vi "PAHS Main.vi"() -> ()   [LabVIEW 2016]
uses:
  Libraries/Controls/Aux CO2 Diags.ctl
  Libraries/Controls/Aux CO2 Selector.ctl
  Libraries/Controls/Processed Variables.ctl
  Libraries/Controls/AirPump Controls.ctl
  Libraries/Controls/Hobbs Meter.ctl
  Libraries/Controls/DAQ Needed.ctl
  Libraries/Controls/IE Ratio knob.ctl
  Libraries/Controls/UI Settings.ctl
  Libraries/Controls/Aux CO2 Control.ctl
  Libraries/Controls/Serial Visa Control.ctl
  Libraries/Controls/Aux TE Control.ctl
  Libraries/Controls/Queues And Others.ctl
  Libraries/Controls/Temperature Cycle.ctl
  Libraries/Controls/Temperature Source.ctl
  <vilib>/Platform/TimedLoop/XDataNode/timing_clust.ctl
  <vilib>/Platform/TimedLoop/XDataNode/nitl_modes.ctl
  <vilib>/Platform/TimedLoop/XDataNode/wakeup.ctl
  Libraries/Miscellaneous/Globals.vi
  <vilib>/platform/TimedLoop/XDataNode/XDataNode.xnode
  <vilib>/Platform/TimedLoop/XDataNode/XDNodeRunTimeDep.lvlib
panel:
  in  "RunTime Mode Settings  2":T1={"Resp Rate Brpm "=0.0, "I:E Ratio"=6, "Insp. Gas Tank"=0, "Exp. Gas Tank"=7} {"Exp. Gas Tank" items=["", "0.000", "0.000", "0.000", "0.000", "0.000", "0.000", "0.000"]; "Insp. Gas Tank" items=["", "0.000", "0.000", "0.000", "0.000", "0.000", "0.000", "0.000"]; "I:E Ratio" max=7 step=1 scale=0.0..7.0; "Resp Rate Brpm" min=0 max=30 step=1 format="%.2f"}
  in  "Cluster 12":T2 {"DAC Setting (ma)" max=1023.0 step=1.0 format="%.2g"; "DAC Setting" max=1023 step=1 format="%02x"}
  out "Status Lights":T3
  in  "Daq Needed":T4 {"Current Settings"."Pump" items=["Pump 0", "Pump 1", "Pump 2", "Pump 3", "Pump 4", "Pump 5"]; "Current Settings"."Chart X axis Timescale" min=20 max=180 step=1; "Current Settings"."RunTime Mode Settings"."Exp. Gas Tank" items=["0.07", "0.031", "0.877", "1.863", "3.881", "5.790", "7.688", "6.000"]; "Current Settings"."RunTime Mode Settings"."Insp. Gas Tank" items=["0.07", "0.031", "0.877", "1.863", "3.881", "5.790", "7.688", "6.000"]; "Current Settings"."RunTime Mode Settings"."I:E Ratio" max=30 scale=0.0..7.0; "Current Settings"."RunTime Mode Settings"."Resp Rate Brpm" min=0 max=30 format="%.2f"; "Current Settings"."TE#2 Configuration"."Serial Port"."XOFF Char" format="%.0x"; "Current Settings"."TE#2 Configuration"."Serial Port"."XON Char" format="%.0x"; "Current Settings"."TE#2 Configuration"."Serial Port"."flow control" items=["None"=0, "XON/XOFF"=1, "RTS/CTS"=2, "DTR/DSR"=4]; "Current Settings"."TE#2 Configuration"."Serial Port"."stop bits" items=["1.0"=10, "1.5"=15, "2.0"=20]; "Current Settings"."TE#2 Configuration"."Serial Port"."data bits" min=5 max=8 step=1; "Current Settings"."TE#2 Configuration"."Serial Port"."baud rate" items=["75"=75, "110"=110, "134"=134, "150"=150, "300"=300, "600"=600, "1200"=1200, "1800"=1800, "2400"=2400, "4800"=4800, "7200"=7200, "9600"=9600, "14400"=14400, "19200"=19200, "28800"=28800, "38400"=38400, "56000"=56000, "57600"=57600, "115200"=115200, "128000"=128000, "230400"=230400]; "Current Settings"."TE#2 Configuration"."Serial Port"."termination char" format="%.0x"; "Current Settings"."TE#1 Configuration"."Serial Port"."XOFF Char" format="%.0x"; "Current Settings"."TE#1 Configuration"."Serial Port"."XON Char" format="%.0x"; "Current Settings"."TE#1 Configuration"."Serial Port"."flow control" items=["None"=0, "XON/XOFF"=1, "RTS/CTS"=2, "DTR/DSR"=4]; "Current Settings"."TE#1 Configuration"."Serial Port"."stop bits" items=["1.0"=10, "1.5"=15, "2.0"=20]; "Current Settings"."TE#1 Configuration"."Serial Port"."data bits" min=5 max=8 step=1; "Current Settings"."TE#1 Configuration"."Serial Port"."baud rate" items=["75"=75, "110"=110, "134"=134, "150"=150, "300"=300, "600"=600, "1200"=1200, "1800"=1800, "2400"=2400, "4800"=4800, "7200"=7200, "9600"=9600, "14400"=14400, "19200"=19200, "28800"=28800, "38400"=38400, "56000"=56000, "57600"=57600, "115200"=115200, "128000"=128000, "230400"=230400]; "Current Settings"."TE#1 Configuration"."Serial Port"."termination char" format="%.0x"; "Current Settings"."Capnometer Configuration"."Device" items=["None", "TidalWave", "LoFlow / Canary", "Capnogard"]; "Current Settings"."Capnometer Configuration"."Serial Port"."XOFF Char" format="%.0x"; "Current Settings"."Capnometer Configuration"."Serial Port"."XON Char" format="%.0x"; "Current Settings"."Capnometer Configuration"."Serial Port"."flow control" items=["None"=0, "XON/XOFF"=1, "RTS/CTS"=2, "DTR/DSR"=4]; "Current Settings"."Capnometer Configuration"."Serial Port"."stop bits" items=["1.0"=10, "1.5"=15, "2.0"=20]; "Current Settings"."Capnometer Configuration"."Serial Port"."data bits" min=5 max=8 step=1; "Current Settings"."Capnometer Configuration"."Serial Port"."baud rate" items=["75"=75, "110"=110, "134"=134, "150"=150, "300"=300, "600"=600, "1200"=1200, "1800"=1800, "2400"=2400, "4800"=4800, "7200"=7200, "9600"=9600, "14400"=14400, "19200"=19200, "28800"=28800, "38400"=38400, "56000"=56000, "57600"=57600, "115200"=115200, "128000"=128000, "230400"=230400]; "Current Settings"."Capnometer Configuration"."Serial Port"."termination char" format="%.0x"; "Current Settings"."DAQx Settings"."Analog Output Settings (Volts)" format="%#.3g"; "Current Settings"."DAQx Settings"."Duty Cycle" min=10.0 max=90.0 format="%.1g"; "Current Settings"."DAQx Settings"."Frequency" min=20.0 max=200.0; "Current Settings"."DataLogging Settings"."Data File Duration (Minutes)" min=2 max=200 format="%#.2g"; "Current Settings"."Calibration Settings"."Tolerance #2" min=2 max=4096; "Current Settings"."Calibration Settings"."Cal. Average" min=2 max=4096; "Current Settings"."Test Settings"."Test Sensor ID" items=["(select)", "RB", "YC", "", "Other"]}
  out "InitializeFile":bool caption="Reset"
  out "Ready":bool caption="Saving Data"
  out "Saving":bool
  in  "Prefix":string
  out "Humidity Error":bool
  out "BD":i32
  in  "breath start time":u32
  out "Raws":T12 {"Chamber Temperature" format="%.2f"; "Ambient Temperature" format="%.2f"; "Bath Temperature" format="%.2f"; "Det. Temperature" format="%.2f"; "Detector Chl 4" format="%.2g"; "Detector Chl 3" format="%.2g"; "Ref CO2" format="%.2g"; "Detector Chl 2" format="%.2g"; "Film Temperature" format="%.2f"; "Humidity" format="%.2f"; "Detector Chl 1" format="%.2g"}
  in  "Raw DAQ Channels 2":cluster{"String":string, "Value":sgl[]}[](array[cluster])=[{"String"="Detector Chnl 1", "Value"=[10.2235565]}, {"String"="Detector Chnl 2", "Value"=[10.219611]}, {"String"="Detector Chnl 3", "Value"=[10.215665]}, {"String"="Detector Chnl 4", "Value"=[10.196594]}, {"String"="CH AI1 - Temp", "Value"=[]}, {"String"="CH AI2 - Temp", "Value"=[]}, {"String"="CH AI3 - (spare)", "Value"=[]}, {"String"="CH AI4 - (spare)", "Value"=[]}, {"String"="CH AI5 - (spare)", "Value"=[]}, {"String"="CH AI6 - PHAvset", "Value"=[]}, {"String"="CH AI7 - PHBvset", "Value"=[]}, {"String"="CH AI8 - PHCvset", "Value"=[]}, {"String"="CH AI9 - PHDvset", "Value"=[]}] {"Value" format="%7.3f"}
  out "start mS time":u32
  in  "Insp Tank":u8
  out "sequence":i64[](array[numeric])
  out "TE Data":sgl[][](array[numeric]) format="%.2g"
  out "Exp Tank":u8
  in  "ExitProgram":bool
  out "Tab Control":T13(tab)
  out "Saving Data":bool
  in  "HomeMode":T14(tab) caption="Status"
  in  "Open Cal":bool
  in  "Store_Cal":bool
  out "Time Since last Zero":u32 format="%<%H:%M:%S>t"
  out "Time Since last Cal":u32 format="%<%H:%M:%S>t"
  in  "Record Button":bool
  out "Saving File":path
  out "starttime":u32
  in  "Zero 2":bool
  in  "Last Calibration":T15
  out "Monitoring Time since last Zero":dbl format="%<%H:%M:%S>t"
  in  "Cluster 3":T17={"pk"=0.0, "RawCO2"=0.0, "Uncal'd"=0.0, "Avg_Hum"=0.0, "Avg'd CO2"=0.0, "Home_CO2"=0.0, "Home_Ref"=0.0, "Home_Hum"=0.0, " Home Temp"=0.0, "Pump Flow Rate"=50, "I:E Ratio"=6, "Brpm"=6.0, "Sim Breaths"=FALSE, "GasTank"=0} {"Brpm" format="%#_2g"; "I:E Ratio" max=7 step=1 scale=0.0..7.0; "Pump Flow Rate" min=50 max=650 step=10 scale=50.0..650.0; "Home Temp" format="%.1f"; "Home_Hum" format="%.1f"; "Home_Ref" format="%.2g"; "Home_CO2" format="%.2g"; "Avg'd CO2" format="%.1g"; "Avg_Hum" format="%.1f"; "Uncal'd" format="%.1g"; "RawCO2" format="%.2g"; "pk" format="%.1g"}
  out "Zero Status":u16(ring)
  out "target":dbl=0.001
  out "standard deviation":u8(slide) scale=1.0..99.0
  out "zcount":i32(slide)=200 scale=0.0..500.0
  out "raws(V)":sgl[](array[numeric])
  out "Capnogram":dbl[][](graph)
  in  "Off":bool
  in  "Cal Required":bool
  in  "Zero Required":bool
  in  "Cluster 8":T18={"Display Uncal'd"=FALSE, "Display Ref"=FALSE, "Ch 1"=FALSE, "Ch 2"=FALSE, "Ch 3"=FALSE, "Ch 4"=TRUE}
  in  "Cluster 7":T19 {"Time Remaining" format="%<%H:%M:%S>t"; "File Duration" format="%<%H:%M:%S>t"}
  out "Char Notice":string="NOT AVAILABLE IN CHARACTERIZATION MODE"
  out "CalTab":enum32{"Page 2", "Page 1"}(tab)
  in  "Cluster 6":T21 {"Time" format="%<%H:%M:%S>t"; "Stable Counter" format="%<%H:%M:%S>t"; "Actual" format="%.2g"; "Set Temp" format="%#.2g"}
  in  "Cluster 5":T22={"ETCO2 %"=0.0, "RR (brpm)"=0.0, "Inhale Time"=0.0, "Exhale Time"=0.0, "Enable Simulated Breaths"=FALSE, "Use Channel"=4} {"Use Channel" min=1 max=4; "RR (brpm)" format="%#.1f"; "ETCO2 %" format="%.1f"}
  out "Waveform Chart 2":dbl[][](graph) caption="Waveform Chart"
  out "Waveform Chart":dbl[][](graph)
  in  "Waveforms":T23={"WaveformA1"=enum."CO2 Ch1", "WaveformA1"=enum."CO2 Ch2", "WaveformA1"=enum."CO2 Ch3", "WaveformA1"=enum."CO2 Ch4", "WaveformA1"=enum."Temp", "WaveformA1"=enum."Humidity", "WaveformA1"=enum."Ref CO2", "WaveformA1"=enum."TE 1&2"}
  out "Gas Tank#":u16(ring) items=["0.07", "0.030", "0.877", "1.863", "3.881", "5.900", "7.688", "6.000", "<OFF>"]
  out "Loflo Status":T24(ring)
  out "Film Sample Name":string
  out "Tank":bool[](array[boolean])
  out "Cluster 4":T25 {"Chamber C" format="%.2f"; "Ambient" format="%.2f"; "Det. `C" format="%.2f"; "Bath `C" format="%.2f"; "Film `C" format="%.2f"; "TE #2" format="%.2f"; "TE #1" format="%.2f"; "Humidity" format="%.2f"; "Ref CO2" format="%.2g"}
  out "Detector Channels":T26 {"Chl 4 (V)" format="%.3g"; "Chl 3 (V)" format="%.3g"; "Chl 2 (V)" format="%.3g"; "Chl 1 (V)" format="%.3g"; "CO2% (4)" format="%.2g"; "CO2% (3)" format="%.2g"; "CO2% (2)" format="%.2g"; "CO2% (1)" format="%.2g"}
  in  "Cluster 9":T27 {"Sensor Under Test" items=["(select)", "RB", "YC", "", "Other"]}
  in  "Cluster 2":T29={" Chamber Temp"=0.0, "Source"=enum."PCB (AI1)", "Bath Source"=TRUE} {"Chamber Temp" format="%.2f"}
  in  "Logging":T30={"Data File Path"=path "c:/data", "Log Filename"=path "", "Data File Duration (Minutes)"=2.0} {"Data File Duration (Minutes)" min=2 max=200 format="%#.2g"}
  out "Pump":u16(ring) items=["Pump 0", "Pump 1", "Pump 2", "Pump 3", "Pump 4", "Pump 5"]
  out "Pump Meter Use (mins)":T31 {"secs" format="%01d"; "mins" format="%01d"}
  in  "Offset Adjust":bool=TRUE
  out "DAC return":sgl[](array[numeric]) caption="Return" format="%.4f"
  out "System #":string
  in  "LEDsON":bool=TRUE
  out "main loop rate":sgl caption="Hz"
  in  "Humidifier":bool=TRUE
  in  "SetDac Button":bool
  in  "Zero":bool
  out "Ticks Interval Time":dbl(graph)
  out "TE Ports":T32 {"ProcessedData" format="%.2g"}
  out "Aux CO2 Port":T33={"Port"="", "Source"=0, "Active"=FALSE, "Baro Pressure"=760, "SerialRxBuffer"="", "Raw CO2 (Torr)"=5.0, "bytes read"=5, "Status"=[], "Status Message"=enum.""} {"Status" format="%x"; "Raw CO2 (Torr)" format="%.2f"; "Baro Pressure" min=400 max=800; "Source" items=["None", "TidalWave", "LoFlow / Canary", "Capnogard"]}
  out "stored time":dbl format="%<%H:%M:%S>t"
  out "stop time":timestamp format="%<%H:%M:%S>T"
  out "DAQ Raw Samples":waveform(dbl)(graph)
  out "loop counter":i32
  out "current time":timestamp format="%<%H:%M:%S>T"
  in  "Run":bool
  out "start time":timestamp format="%<%H:%M:%S>T"
  out "Notes":string
  out "Raw (Torr)":sgl=5.0
  out "Digital Output":T34(array[cluster])=[{"Boolean"=TRUE, "String"="PO.0", "String 2"="Test"}, {"Boolean"=FALSE, "String"="PO.1", "String 2"="Dual Channel"}, {"Boolean"=TRUE, "String"="PO.2", "String 2"="Air Pump"}, {"Boolean"=FALSE, "String"="PO.3", "String 2"="Optical Drive"}, {"Boolean"=TRUE, "String"="PO.4", "String 2"="Pulsed Drive"}, {"Boolean"=FALSE, "String"="PO.5", "String 2"="Exp. Phase"}, {"Boolean"=FALSE, "String"="PO.6", "String 2"="/Expiratory"}, {"Boolean"=FALSE, "String"="PO.7", "String 2"="Insp. Phase"}, {"Boolean"=FALSE, "String"="PO.8", "String 2"="/Inspiratory"}, {"Boolean"=TRUE, "String"="PO.9", "String 2"="Gas Tank #0"}, {"Boolean"=FALSE, "String"="PO.10", "String 2"="Gas Tank #1"}, {"Boolean"=FALSE, "String"="PO.11", "String 2"="Gas Tank #2"}, {"Boolean"=FALSE, "String"="PO.12", "String 2"="Gas Tank #3"}, {"Boolean"=FALSE, "String"="PO.13", "String 2"="Gas Tank #4"}, {"Boolean"=FALSE, "String"="PO.14", "String 2"="Gas Tank #5"}, {"Boolean"=FALSE, "String"="PO.15", "String 2"="Gas Tank #6"}, {"Boolean"=FALSE, "String"="PO.16", "String 2"="Gas Tank #7"}, {"Boolean"=FALSE, "String"="PO.17", "String 2"="Solenoid #1"}, {"Boolean"=FALSE, "String"="PO.18", "String 2"="Solenoid #2"}, {"Boolean"=FALSE, "String"="PO.19", "String 2"="(spare)"}, {"Boolean"=FALSE, "String"="PO.20", "String 2"="(spare)"}, {"Boolean"=FALSE, "String"="PO.21", "String 2"="(spare)"}, {"Boolean"=FALSE, "String"="PO.22", "String 2"="(spare)"}, {"Boolean"=FALSE, "String"="PO.23", "String 2"="(spare)"}, {"Boolean"=FALSE, "String"="PO.24", "String 2"="(spare)"}, {"Boolean"=FALSE, "String"="PO.25", "String 2"="(spare)"}, {"Boolean"=FALSE, "String"="PO.26", "String 2"="(spare)"}, {"Boolean"=FALSE, "String"="PO.27", "String 2"="(spare)"}, {"Boolean"=FALSE, "String"="PO.28", "String 2"="(spare)"}, {"Boolean"=FALSE, "String"="PO.29", "String 2"="(spare)"}, {"Boolean"=FALSE, "String"="PO.30", "String 2"="(spare)"}, {"Boolean"=FALSE, "String"="PO.31", "String 2"="(spare)"}]
  in  "Set Point1":sgl format="%#.1f"
  in  "Set Point2":sgl format="%#.1f"
  out "Set Point Changed":bool
  out "Raw DAQ Channels":cluster{"String":string, "Value":sgl[]}[](array[cluster])=[{"String"="Detector Chnl 1", "Value"=[10.2235565]}, {"String"="Detector Chnl 2", "Value"=[10.219611]}, {"String"="Detector Chnl 3", "Value"=[10.215665]}, {"String"="Detector Chnl 4", "Value"=[10.196594]}, {"String"="CH AI1 - Temp", "Value"=[]}, {"String"="CH AI2 - Temp", "Value"=[]}, {"String"="CH AI3 - (spare)", "Value"=[]}, {"String"="CH AI4 - (spare)", "Value"=[]}, {"String"="CH AI5 - (spare)", "Value"=[]}, {"String"="CH AI6 - PHAvset", "Value"=[]}, {"String"="CH AI7 - PHBvset", "Value"=[]}, {"String"="CH AI8 - PHCvset", "Value"=[]}, {"String"="CH AI9 - PHDvset", "Value"=[]}] {"Value" format="%7.3f"}
  out "Actual dt":dbl format="%0.6f"
  out "DAC Setting":u16[](array[numeric]) format="%x"
  out "last cal time":timestamp format="%<%H:%M:%S>T"
  out "last zero time":timestamp format="%<%H:%M:%S>T"
  in  "Whole Pulse":bool=TRUE
  out "Loflo":bool
  out "digital  out":u32 format="%08x"
  out "Sequence Count":i32
  out "Baro Pressure":u16=760 min=400 max=800
  out "DAC current 2":sgl[](array[numeric]) caption="DAC" format="%.4f"
  in  "AirPump Controls":T35={"Air Pump PWM"=99.9, "Solenoid #1"=FALSE, "Solenoid #2"=FALSE, "Air Pump On"=FALSE, "Short tubing"=FALSE, "Loflo Connected"=FALSE, "Flow(ml)"=0, "Wait Active"=FALSE} {"Air Pump PWM" min=0 max=99.9 scale=0.0..99.9 scale format="%.1f"}
  in  "+":bool
  in  "-":bool
  out "?":T36 {"LED offtime (mS)" format="%#.3f"; "LED ontime (mS)" format="%#.3f"}
  out "Cluster":T37={"DAQ Device Ind."="", "ProductCategory"=14643, "ProductType"="", "ProductNum"=0, "DevSerialNum"=0} {"ProductCategory" items=["M Series DAQ"=14643, "X Series DAQ"=15858, "E Series DAQ"=14642, "S Series DAQ"=14644, "B Series DAQ"=14662, "SC Series DAQ"=14645, "USB DAQ"=14646, "AO Series"=14647, "Digital I/O"=14648, "TIO Series"=14661, "Dynamic Signal Acquisition"=14649, "Switches"=14650, "CompactDAQ Chassis"=14658, "C Series Module"=14659, "SCXI Module"=14660, "SCC Connector Block"=14704, "SCC Module"=14705, "NI ELVIS"=14755, "Network DAQ"=14829, "SC Express"=15886, "Unknown"=12588]}
  out "Application Info":T38={"SW Phase"="Phase II", "SW Revision"="P2-1.0.2", "Build Time / Date"=timestamp(3498222600 s since 1904-01-01), "Config Path"=path ""} {"Build Time / Date" format="%<%H:%M\n%m/%d/%Y>T"}
  # "Hidden Variables"
  # "Note: Setting Brpm to zero will\ndisable Insp / Exp digital output."
  # "Note: Setting Brpm to zero will\ndisable Insp / Exp digital output."
  # "mmHg"
  # "pts"
  # "tolerance"
  # "AN5 (Temp 1)"
  # "AN6 (Temp 2)"
  # "AN7 (Temp 3)"
  # "AN8 (T FET)"
  # "AN0 (T POT)"
  # "Tref (Set Pt))"
  # "(Spare)"
  # "%"
  # "DAQMx In Use |"
  # "Program Running |"
  # "PWM Active & OK |"
  # "Main Loop Active |"
  # "(Volts)"
  # "DAQ Properties"
  # "Currents (A)"
  # "Nudge SP1"
  # "AN5 (Temp 1)"
  # "AN6 (Temp 2)"
  # "AN7 (Temp 3)"
  # "AN8 (T FET)"
  # "AN0 (T POT)"
  # "Tref (Set Pt))"
  # "(Spare)"
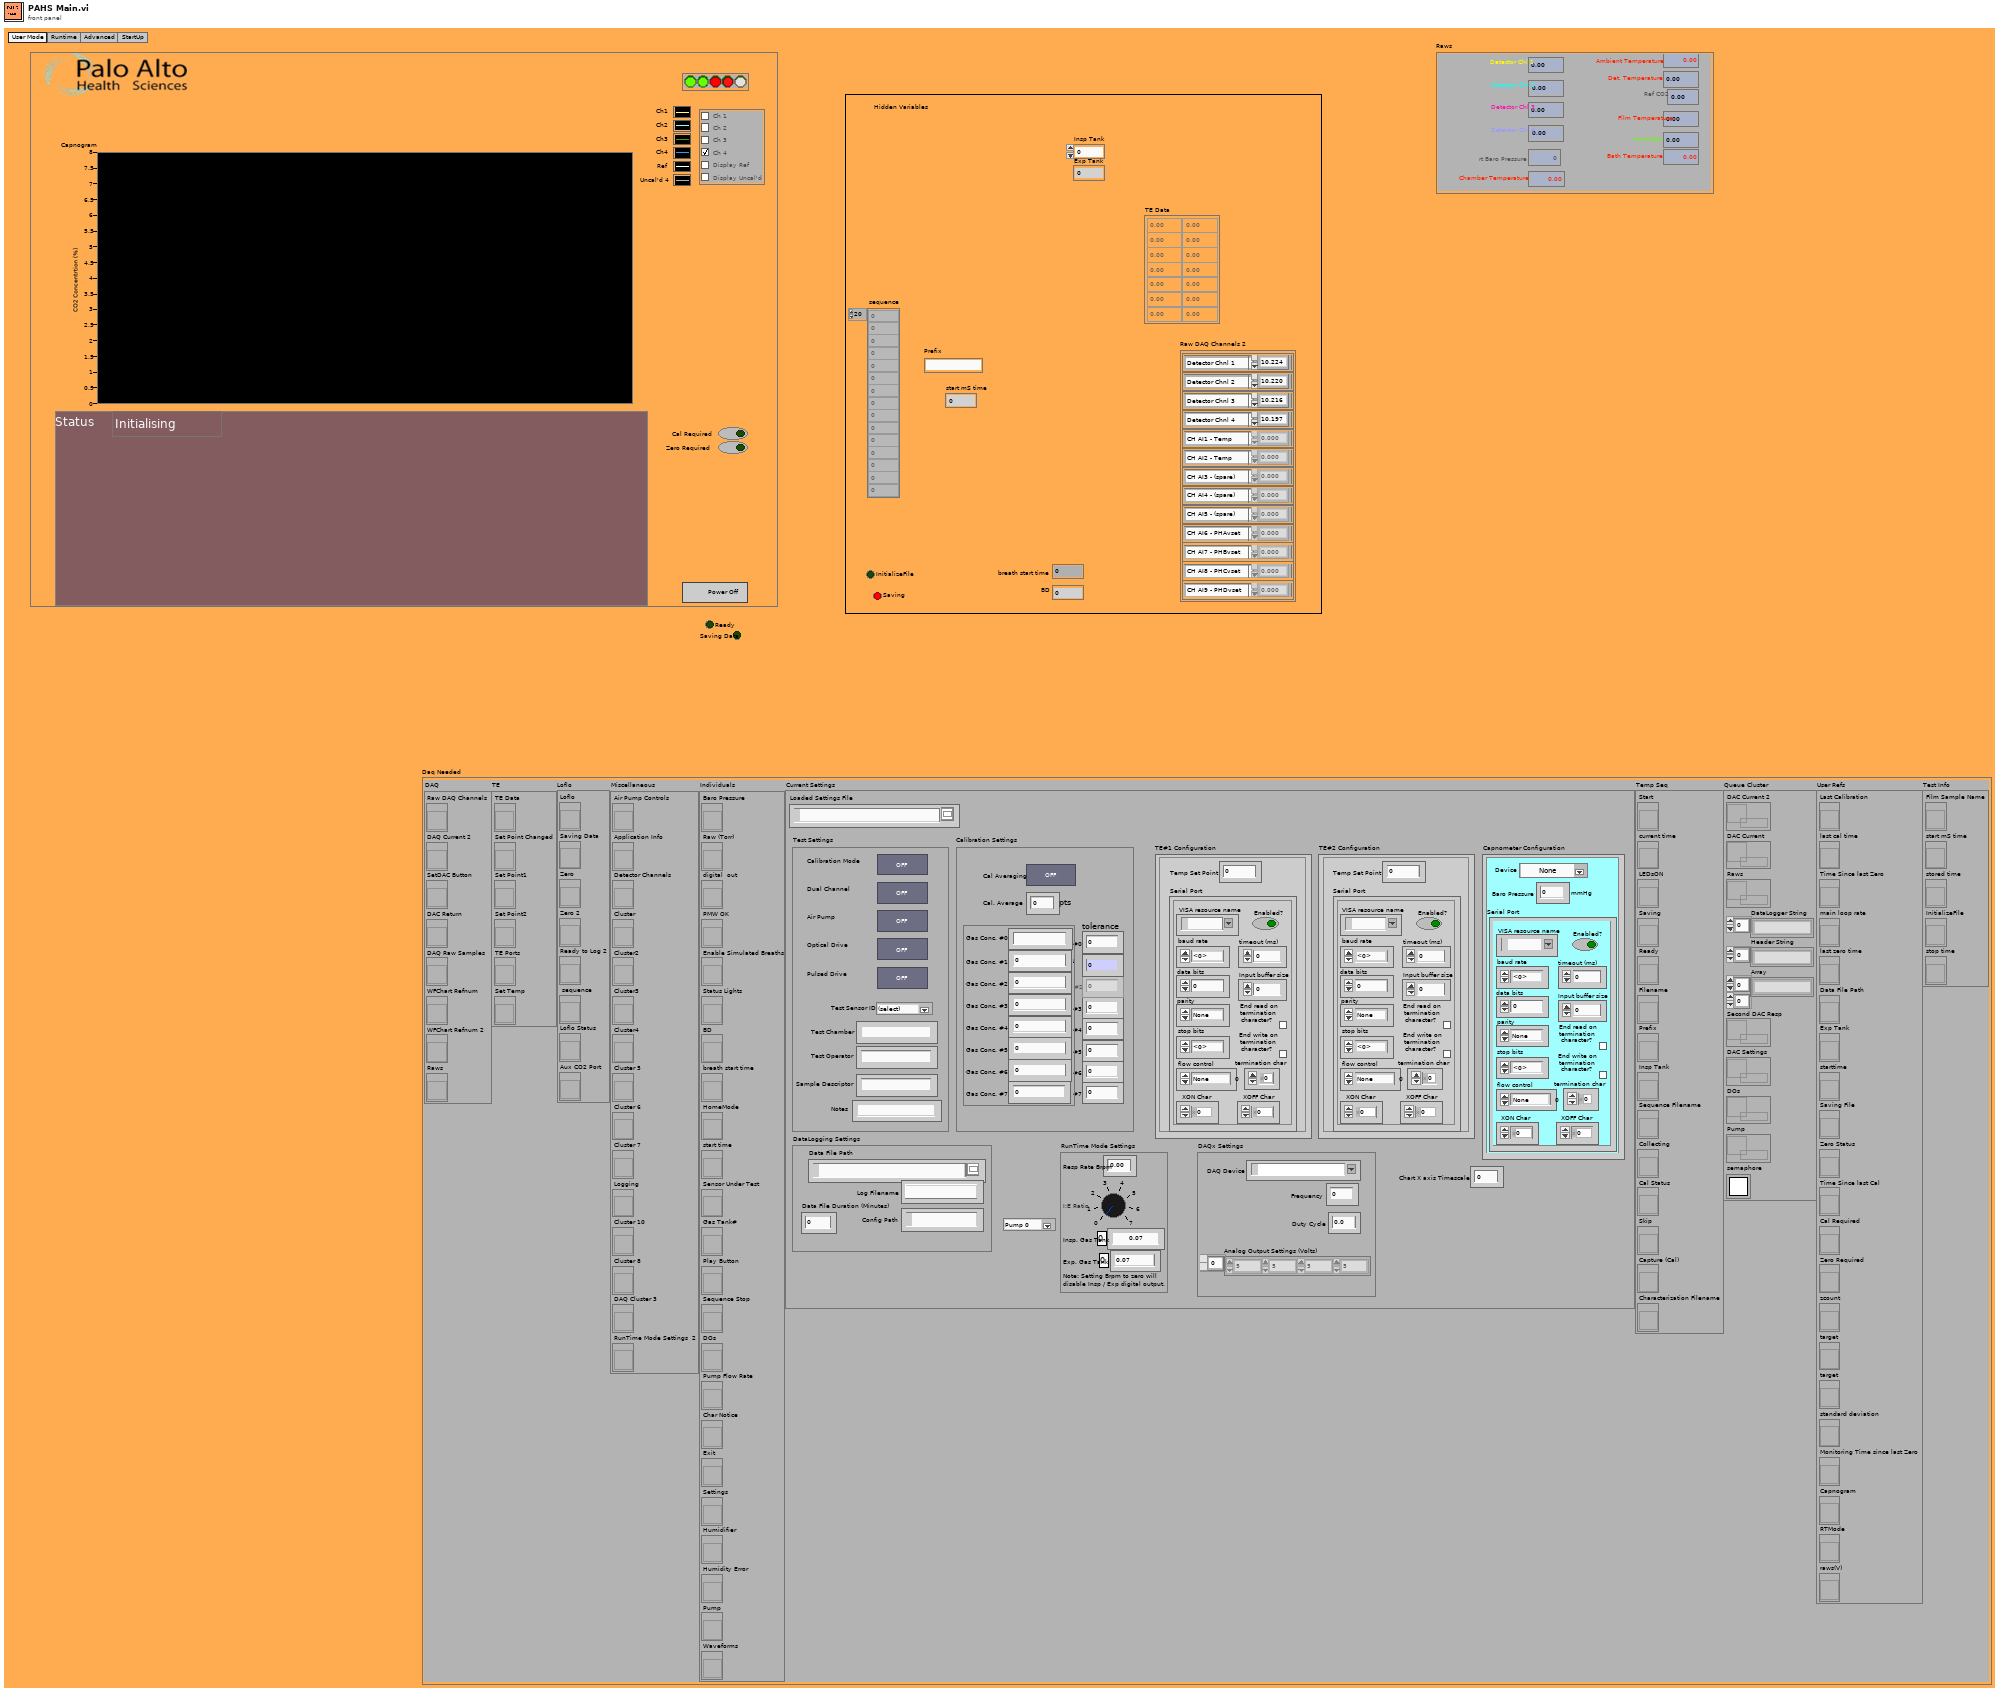
[diagram p1: front panel]
types:
  T1 = cluster{"Resp Rate Brpm ":sgl, "I:E Ratio":u8, "Insp. Gas Tank":u16, "Exp. Gas Tank":u16}
  T2 = cluster{"DAC Setting":u16[], "DAC Setting (ma)":dbl[]}
  T3 = cluster{"InUserMode":bool, "SimMode":bool, "Loop Active":bool, "PWM OK":bool, "Running":bool}
  T4 = typedef "DAQ Needed.ctl" = cluster{"DAQ":cluster{"Raw DAQ Channels":refnum<vi>, "DAQ Current 2":refnum<vi>, "SetDAC Button":refnum<vi>, "DAC Return":refnum<vi>, "DAQ Raw Samples":refnum<vi>, "WFChart Refnum":refnum<vi>, "WFChart Refnum 2":refnum<vi>, "Raws":refnum<vi>}, "TE":cluster{"TE Data":refnum<vi>, "Set Point Changed":refnum<vi>, "Set Point1":refnum<vi>, "Set Point2":refnum<vi>, "TE Ports":refnum<vi>, "Set Temp":refnum<vi>}, "Loflo":cluster{"Loflo":refnum<vi>, "Saving Data":refnum<vi>, "Zero":refnum<vi>, "Zero 2":refnum<vi>, "Ready to Log 2":refnum<vi>, " sequence":refnum<vi>, "Loflo Status ":refnum<vi>, "Aux CO2 Port":refnum<vi>}, "Miscellaneous":cluster{"Air Pump Controls":refnum<vi>, "Application Info":refnum<vi>, "Detector Channels ":refnum<vi>, "Cluster":refnum<vi>, "Cluster2":refnum<vi>, "Cluster3":refnum<vi>, "Cluster4":refnum<vi>, "Cluster 5":refnum<vi>, "Cluster 6":refnum<vi>, "Cluster 7":refnum<vi>, "Logging":refnum<vi>, "Cluster 10":refnum<vi>, "Cluster 8":refnum<vi>, "DAQ Cluster 3":refnum<vi>, "RunTime Mode Settings  2":refnum<vi>}, "Individuals":cluster{"Baro Pressure":refnum<vi>, "Raw (Torr)":refnum<vi>, "digital  out":refnum<vi>, "PMW OK":refnum<vi>, "Enable Simulated Breaths":refnum<vi>, "Status Lights":refnum<vi>, "BD":refnum<vi>, "breath start time":refnum<vi>, "HomeMode":refnum<vi>, "start time":refnum<vi>, "Sensor Under Test":refnum<vi>, "Gas Tank#":refnum<vi>, "Play Button":refnum<vi>, "Sequence Stop":refnum<vi>, "DOs":refnum<vi>, "Pump Flow Rate":refnum<vi>, "Char Notice":refnum<vi>, "Exit":refnum<vi>, "Settings":refnum<vi>, "Humidifier":refnum<vi>, "Humidity Error":refnum<vi>, "Pump":refnum<vi>, "Waveforms":refnum<vi>}, "Current Settings":T5, "Temp Seq":cluster{"Start":refnum<vi>, "current time":refnum<vi>, "LEDsON":refnum<vi>, "Saving":refnum<vi>, "Ready":refnum<vi>, "Filename":refnum<vi>, "Prefix":refnum<vi>, "Insp Tank":refnum<vi>, "Sequence Filename":refnum<vi>, "Collecting":refnum<vi>, "Cal Status":refnum<vi>, "Skip":refnum<vi>, "Capture (Cal)":refnum<vi>, "Characterization Filename":refnum<vi>}, "Queue Cluster":T10, "User Refs":cluster{"Last Calibration":refnum<vi>, "last cal time":refnum<vi>, "Time Since last Zero":refnum<vi>, "main loop rate":refnum<vi>, "last zero time":refnum<vi>, "Data File Path":refnum<vi>, "Exp Tank":refnum<vi>, "starttime":refnum<vi>, "Saving File":refnum<vi>, "Zero Status":refnum<vi>, "Time Since last Cal":refnum<vi>, "Cal Required":refnum<vi>, "Zero Required":refnum<vi>, "zcount":refnum<vi>, "target":refnum<vi>, "target":refnum<vi>, "standard deviation":refnum<vi>, "Monitoring Time since last Zero":refnum<vi>, "Capnogram":refnum<vi>, "RTMode":refnum<vi>, "raws(V)":refnum<vi>}, "Test Info":cluster{"Film Sample Name":refnum<vi>, "start mS time":refnum<vi>, "stored time":refnum<vi>, "InitializeFile":refnum<vi>, "stop time":refnum<vi>}}
  T5 = typedef "UI Settings.ctl" = cluster{"Loaded Settings File":path, "Test Settings":cluster{"Dual Channel":bool, "Air Pump":bool, "Optical Drive":bool, "Pulsed Drive":bool, "Calibration Mode":bool, "Test Sensor ID":u16, "Test Chamber":string, "Test Operator":string, "Sample Descriptor":string, "Notes":string}, "Calibration Settings":cluster{"Cal. Average":u16, "Cal Averaging":bool, "Tolerance #0":sgl, "Tolerance #7":sgl, "Tolerance #6":sgl, "Tolerance #5":sgl, "Tolerance #4":sgl, "Tolerance #3":sgl, "Tolerance #2":sgl, "Tolerance #1":sgl, "Gas Tank Settings":cluster{"Gas Conc. #0":string, "Gas Conc. #1":sgl, "Gas Conc. #2":sgl, "Gas Conc. #3":sgl, "Gas Conc. #4":sgl, "Gas Conc. #5":sgl, "Gas Conc. #6":sgl, "Gas Conc. #7":sgl}}, "DataLogging Settings":cluster{"Data File Path":path, "Data File Duration (Minutes)":sgl, "Log Filename":string, "Config Path":path}, "DAQx Settings":cluster{"DAQ Device":tag, "Frequency":dbl, "Duty Cycle":dbl, "Analog Output Settings (Volts)":sgl[]}, "Capnometer Configuration":T6, "TE#1 Configuration":T9, "TE#2 Configuration":T9, "RunTime Mode Settings ":cluster{"Resp Rate Brpm ":sgl, "I:E Ratio":u8, "Insp. Gas Tank":u16, "Exp. Gas Tank":u16}, "Chart X axis Timescale":u16, "Pump":u16}
  T6 = typedef "Aux CO2 Control.ctl" = cluster{"Serial Port":T7, "Baro Pressure":u32, "Device":T8}
  T7 = typedef "Serial Visa Control.ctl" = cluster{"termination char":u8, "End read on termination character?":bool, "Enabled?":bool, "VISA resource name":refnum<visa-resource-name>, "baud rate":u32, "data bits":u16, "parity":enum16{"None", "Odd", "Even", "Mark", "Space"}, "stop bits":u16, "flow control":u16, "timeout (ms)":u32, "Input buffer size":u32, "End write on termination character?":bool, "XON Char":u8, "XOFF Char":u8}
  T8 = typedef "Aux CO2 Selector.ctl" = u16
  T9 = typedef "Aux TE Control.ctl" = cluster{"Temp Set Point":sgl, "Serial Port":T7}
  T10 = typedef "Queues And Others.ctl" = cluster{"DAC Current 2":refnum<queue>, "DAC Current":refnum<queue>, "Raws":refnum<queue>, "DataLogger String":string[], "Header String":string[], "Array":string[][], "Second DAC Resp":refnum<queue>, "DAC Settings":refnum<queue>, "DOs":refnum<queue>, "Pump":refnum<queue>, "semaphore":T11}
  T11 = typedef "Semaphore RefNum" = refnum<k1>
  T12 = typedef "Processed Variables.ctl" = cluster{"Detector Chl 1":sgl, "Humidity":dbl, "Film Temperature":dbl, "Detector Chl 2":sgl, "Ref CO2":sgl, "Detector Chl 3":sgl, "Detector Chl 4":sgl, "Det. Temperature":dbl, "Bath Temperature":dbl, "Ambient Temperature":dbl, "rt Baro Pressure":u16, "Chamber Temperature":dbl}
  T13 = enum32{"User Mode", "Runtime", "Advanced", "StartUp"}
  T14 = enum32{"Initialising", "Monitoring", "Calibrate", "Zeroing"}
  T15 = cluster{"Last Cal Date":string, "Last Cal Time":string, "View Cal Details":bool}
  T16 = typedef "IE Ratio knob.ctl" = u8
  T17 = cluster{"pk":sgl, "RawCO2":sgl, "Uncal'd":sgl, "Avg_Hum":sgl, "Avg'd CO2":sgl, "Home_CO2":sgl, "Home_Ref":sgl, "Home_Hum":sgl, " Home Temp":dbl, "Pump Flow Rate":u16, "I:E Ratio":T16, "Brpm":sgl, "Sim Breaths":bool, "GasTank":u8}
  T18 = cluster{"Display Uncal'd":bool, "Display Ref":bool, "Ch 1":bool, "Ch 2":bool, "Ch 3":bool, "Ch 4":bool}
  T19 = cluster{"Start":bool, "Filename":path, "Ready to Log 2":bool, "x = 0?":bool, "File Duration":sgl, "Time Remaining":i16}
  T20 = typedef "Temperature Cycle.ctl" = enum16{"Initializing", "Enter Filenames", "Ready...", "Loading Characterisations", "Storing Temp Profile", "Setting Temperature 1", "Wait to Set Temperature 2", "Waiting for Stablization", "Thermal Soak", "Starting Sequence", "Collecting", "Storing Data", "Terminating", "Characterisation Complete"}
  T21 = cluster{"Characterisation Filename":path, "Sequence Filename":path, "Set Temp":sgl, "Actual":sgl, "Capture (Cal)":bool, "Stable Counter":u32, "Time":u32, "Step":u16, "of":u16, "InRange":bool, "Cal Status":T20, "Collecting":bool, "Saved":bool, "Skip":bool}
  T22 = cluster{"ETCO2 %":sgl, "RR (brpm)":sgl, "Inhale Time":sgl, "Exhale Time":sgl, "Enable Simulated Breaths":bool, "Use Channel":u8}
  T23 = cluster{"WaveformA1":enum16{"<OFF>", "CO2 Ch1"}, "WaveformA1":enum16{"<OFF>", "CO2 Ch2"}, "WaveformA1":enum16{"<OFF>", "CO2 Ch3"}, "WaveformA1":enum16{"<OFF>", "CO2 Ch4"}, "WaveformA1":enum16{"<OFF>", "Temp"}, "WaveformA1":enum16{"<OFF>", "Humidity"}, "WaveformA1":enum16{"<OFF>", "Ref CO2"}, "WaveformA1":enum16{"<OFF>", "TE 1&2", "TE #1", "TE #2"}}
  T24 = enum16{"", "Sensor Over Temp", "Sensor Faulty", "Set BaroP", "Capno in Sleep Mode", "Zero In Progress", "Sensor Warm Up", "Check Sampling Line", "Zero Required", "CO2 Out Of Range", "Check Airway Adapter", "LoFlo Not Connected"}
  T25 = cluster{"Ref CO2":sgl, "Humidity":sgl, "TE #1":sgl, "TE #2":sgl, " Film `C":dbl, "Bath `C":dbl, " Det. `C":dbl, " Ambient":dbl, " Chamber C ":dbl}
  T26 = cluster{"CO2% (1)":sgl, "CO2% (2)":sgl, "CO2% (3)":sgl, "CO2% (4)":sgl, "Chl 1 (V)":sgl, "Chl 2 (V)":sgl, "Chl 3 (V)":sgl, "Chl 4 (V)":sgl}
  T27 = cluster{"RTMode":bool, "Sensor Under Test":u16, "Cluster 2":cluster{"Operator":string, "Chamber":string, "Drive":string, "Channels":string}, "Sequence Stop":bool, "Play Button":bool, "Settings":bool, "Advanced":bool, "Exit":bool}
  T28 = typedef "Temperature Source.ctl" = enum16{"Simulated", "PCB (AI1)", "Film (TE1,2)", "Bath (TE2,2)", "TE1,1 - AN5", "TE2,1 - AN5", "TE1,3 - AN7", "TE2,3 - AN7"}
  T29 = cluster{" Chamber Temp":dbl, "Source":T28, "Bath Source":bool}
  T30 = cluster{"Data File Path":path, "Log Filename":path, "Data File Duration (Minutes)":sgl}
  T31 = typedef "Hobbs Meter.ctl" = cluster{"mins":u8[], "secs":u8[]}
  T32 = cluster{"TE Port 1":refnum<visa-resource-name>, "TE Port 2":refnum<visa-resource-name>, "ProcessedData":sgl[][], "Bytes Read":i16[], "TE OK? 2":bool[]}
  T33 = typedef "Aux CO2 Diags.ctl" = cluster{"Port":refnum<visa-resource-name>, "Source":T8, "Active":bool, "Baro Pressure":u16, "SerialRxBuffer":string, "Raw CO2 (Torr)":sgl, "bytes read":i16, "Status":u8[], "Status Message":enum16{"", "Sensor Over Temp", "Sensor Faulty", "Set BaroP", "Capno in Sleep Mode", "Zero In Progress", "Sensor Warm Up", "Check Sampling Line", "Zero Required", "CO2 Out Of Range", "Check Airway Adapter", "LoFlo Not Connected"}}
  T34 = cluster{"Boolean":bool, "String":string, "String 2":string}[]
  T35 = typedef "AirPump Controls.ctl" = cluster{"Air Pump PWM":sgl, "Solenoid #1":bool, "Solenoid #2":bool, "Air Pump On":bool, "Short tubing":bool, "Loflo Connected":bool, "Flow(ml)":u16, "Wait Active":bool}
  T36 = cluster{"DAQ sampling rate":dbl, "#samples":dbl, "Trigger rate (Hz)":dbl, "LED ontime (mS)":dbl, "LED offtime (mS)":dbl}
  T37 = cluster{"DAQ Device Ind.":tag, "ProductCategory":i32, "ProductType":string, "ProductNum":u32, "DevSerialNum":u32}
  T38 = cluster{"SW Phase":string, "SW Revision":string, "Build Time / Date":timestamp, "Config Path":path}
  T39 = cluster{"SW Phase":string, "SW Revision":string, "Build Time / Date":timestamp}
  T40 = enum16{"Change Item", "Get Value", "Return Count"}
  T41 = enum8{"Enabled", "Disabled", "Disabled and Grayed Out"}
  T42 = typedef "XDNodeRunTimeDep.lvlib/timing_clust.ctl" = cluster{"Expected End [f-1]":u64, "Actual End [f-1]":u64, "Finished Late? [f-1]":bool, "Expected End [i-1]":u64, "Actual End [i-1]":u64, "Finished Late? [i-1]":bool, "Expected Start [i]":u64, "Actual Start [i]":u64, "Expected Start [f]":u64, "Actual Start [f]":u64, "Source Name":string, "Structure Name":string, "Period":i64, "Deadline":i64, "Offset":i64, "Start":i64, "Priority":i32, "Timeout":i32, "Mode":T43, "Wakeup Reason":T44, "Error":errorcluster, "Source Type":string, "Secondary Source Type":string, "Global End Time":u64, "Global Start Time":u64, "Frame Duration":u64, "Iteration Duration":u64, "Assigned CPU":i32, "I/O Scan Engine Mode":u32}
  T43 = typedef "XDNodeRunTimeDep.lvlib/nitl_modes.ctl" = enum32{"No Change", "Process missed periods, maintain original phase", "Discard missed periods, maintain original phase", "Process missed periods, ignore original phase", "Discard missed periods, ignore original phase"}
  T44 = typedef "XDNodeRunTimeDep.lvlib/wakeup.ctl" = enum32{"Normal", "Aborted", "Asynchronous wakeup", "Timing source error", "Timed loop error", "Timeout"}
  T45 = cluster{"Solenoid #1":bool, "Solenoid #2":bool, "Air Pump On":bool, "Flow(ml)":u16}
  T46 = cluster{"Start":refnum<vi>, "current time":refnum<vi>, "LEDsON":refnum<vi>, "Saving":refnum<vi>, "Ready":refnum<vi>, "Filename":refnum<vi>, "Prefix":refnum<vi>, "Insp Tank":refnum<vi>, "Sequence Filename":refnum<vi>, "Collecting":refnum<vi>, "Cal Status":refnum<vi>, "Skip":refnum<vi>, "Capture (Cal)":refnum<vi>, "Characterisation Filename":refnum<vi>}
  T47 = cluster{"Film Sample Name":refnum<vi>, "start mS time":refnum<vi>, "stored time":refnum<vi>, "InitializeFile":refnum<vi>, "stop time":refnum<vi>}
  T48 = cluster{"Header String":string[], "DataLogger String":string[], "Drive":string, "App Info":cluster{"SW Revision":string, "SW Phase":string, "Build Time / Date":timestamp}}
  T49 = cluster{"DAQ Device Ind.":refnum<vi>, "SimMode":refnum<vi>, "I:E Ratio":refnum<vi>}
  T50 = cluster{"#samples":dbl, "DAQ sampling rate":dbl, "LED rate (Hz)":dbl, "Actual dt":dbl, "LED ontime (mS)":dbl, "LED offtime (mS)":dbl}
  T51 = typedef "DAQTasks.ctl" = cluster{"AI_Det_Chnl In":refnum<k21>[], "AI_Task Aux In":refnum<k21>, "Dout_Task In":refnum<k21>, "PWM_Tasks":refnum<k21>[]}
  T52 = cluster{"Actual dt":dbl, "Exp Time":u32, "Loop Rate":dbl, "Tab Control":enum32{"User Mode", "Runtime", "Advanced", "StartUp"}, "Numeric out":u32, "System #":string}
  T53 = cluster{"Avg Hum":dbl, "Humidity":dbl, "Chamber Temperature":dbl, "Ref CO2":sgl, "Array":sgl[], "RawCO2s":dbl[], "ETCO2 Out":dbl, "RR Out":dbl, "BD":i32, bool}
  T54 = typedef "Calibration Coefficients.ctl" = cluster{"CalFile Used":path, "TYPE":string, "DATE":string, "Humidity":sgl, "Chamber Temp":dbl, "CO2_calgas":dbl, "V_(RA,5mA)":dbl, "V_(RA,15mA)":dbl, "mI":dbl, "V_0d_ImA (actual)":dbl, "V_6d_ImA (actual)":dbl, "I_span":dbl, "DAC":u16, "A":dbl, "B":dbl, "C":dbl, "D":dbl, "V6d":dbl, "A'":dbl, "B'":dbl, "C'":dbl, "D'":dbl, "V0d":dbl, "CalDate":string, "CalTime":string, "duration":dbl, "Detector Channel":string, "a2":dbl, "a3":dbl, "a4":dbl, "a5":dbl, "b2":dbl, "c2":dbl, "b3":dbl, "c3":dbl, "b4":dbl, "c4":dbl, "b5":dbl, "c5":dbl, "a7":dbl, "a8":dbl, "a9":dbl, "a10":dbl, "b7":dbl, "b8":dbl, "b9":dbl, "b10":dbl, "c7":dbl, "c8":dbl, "c9":dbl, "c10":dbl, "cal_offs_adj":dbl, "cal_gain_adj":dbl, "C6d":dbl, "C0d":dbl, "Cal_currernt":dbl, "C2V":u16, "V2C":u16, "Zero Date":string, "Zero Time":string, "Number of Zeroes":u16, "V_(()d, average)":dbl, "V_offs ":dbl, "G_adj":dbl, "Pump Flow Rate":u16, "Zero Required? ":bool, "Calibrate Required?":bool, "cal_utc":dbl, "zero_utc":dbl, "Elapsed Time":dbl, "PCB":string, "m0":dbl, "b0":dbl}
  T55 = cluster{"WaveformA1":bool, "WaveformA1":bool, "WaveformA1":bool, "WaveformA1":bool, "WaveformA1":bool, "WaveformA1":bool, "WaveformA1":bool, "WaveformA1":bool}
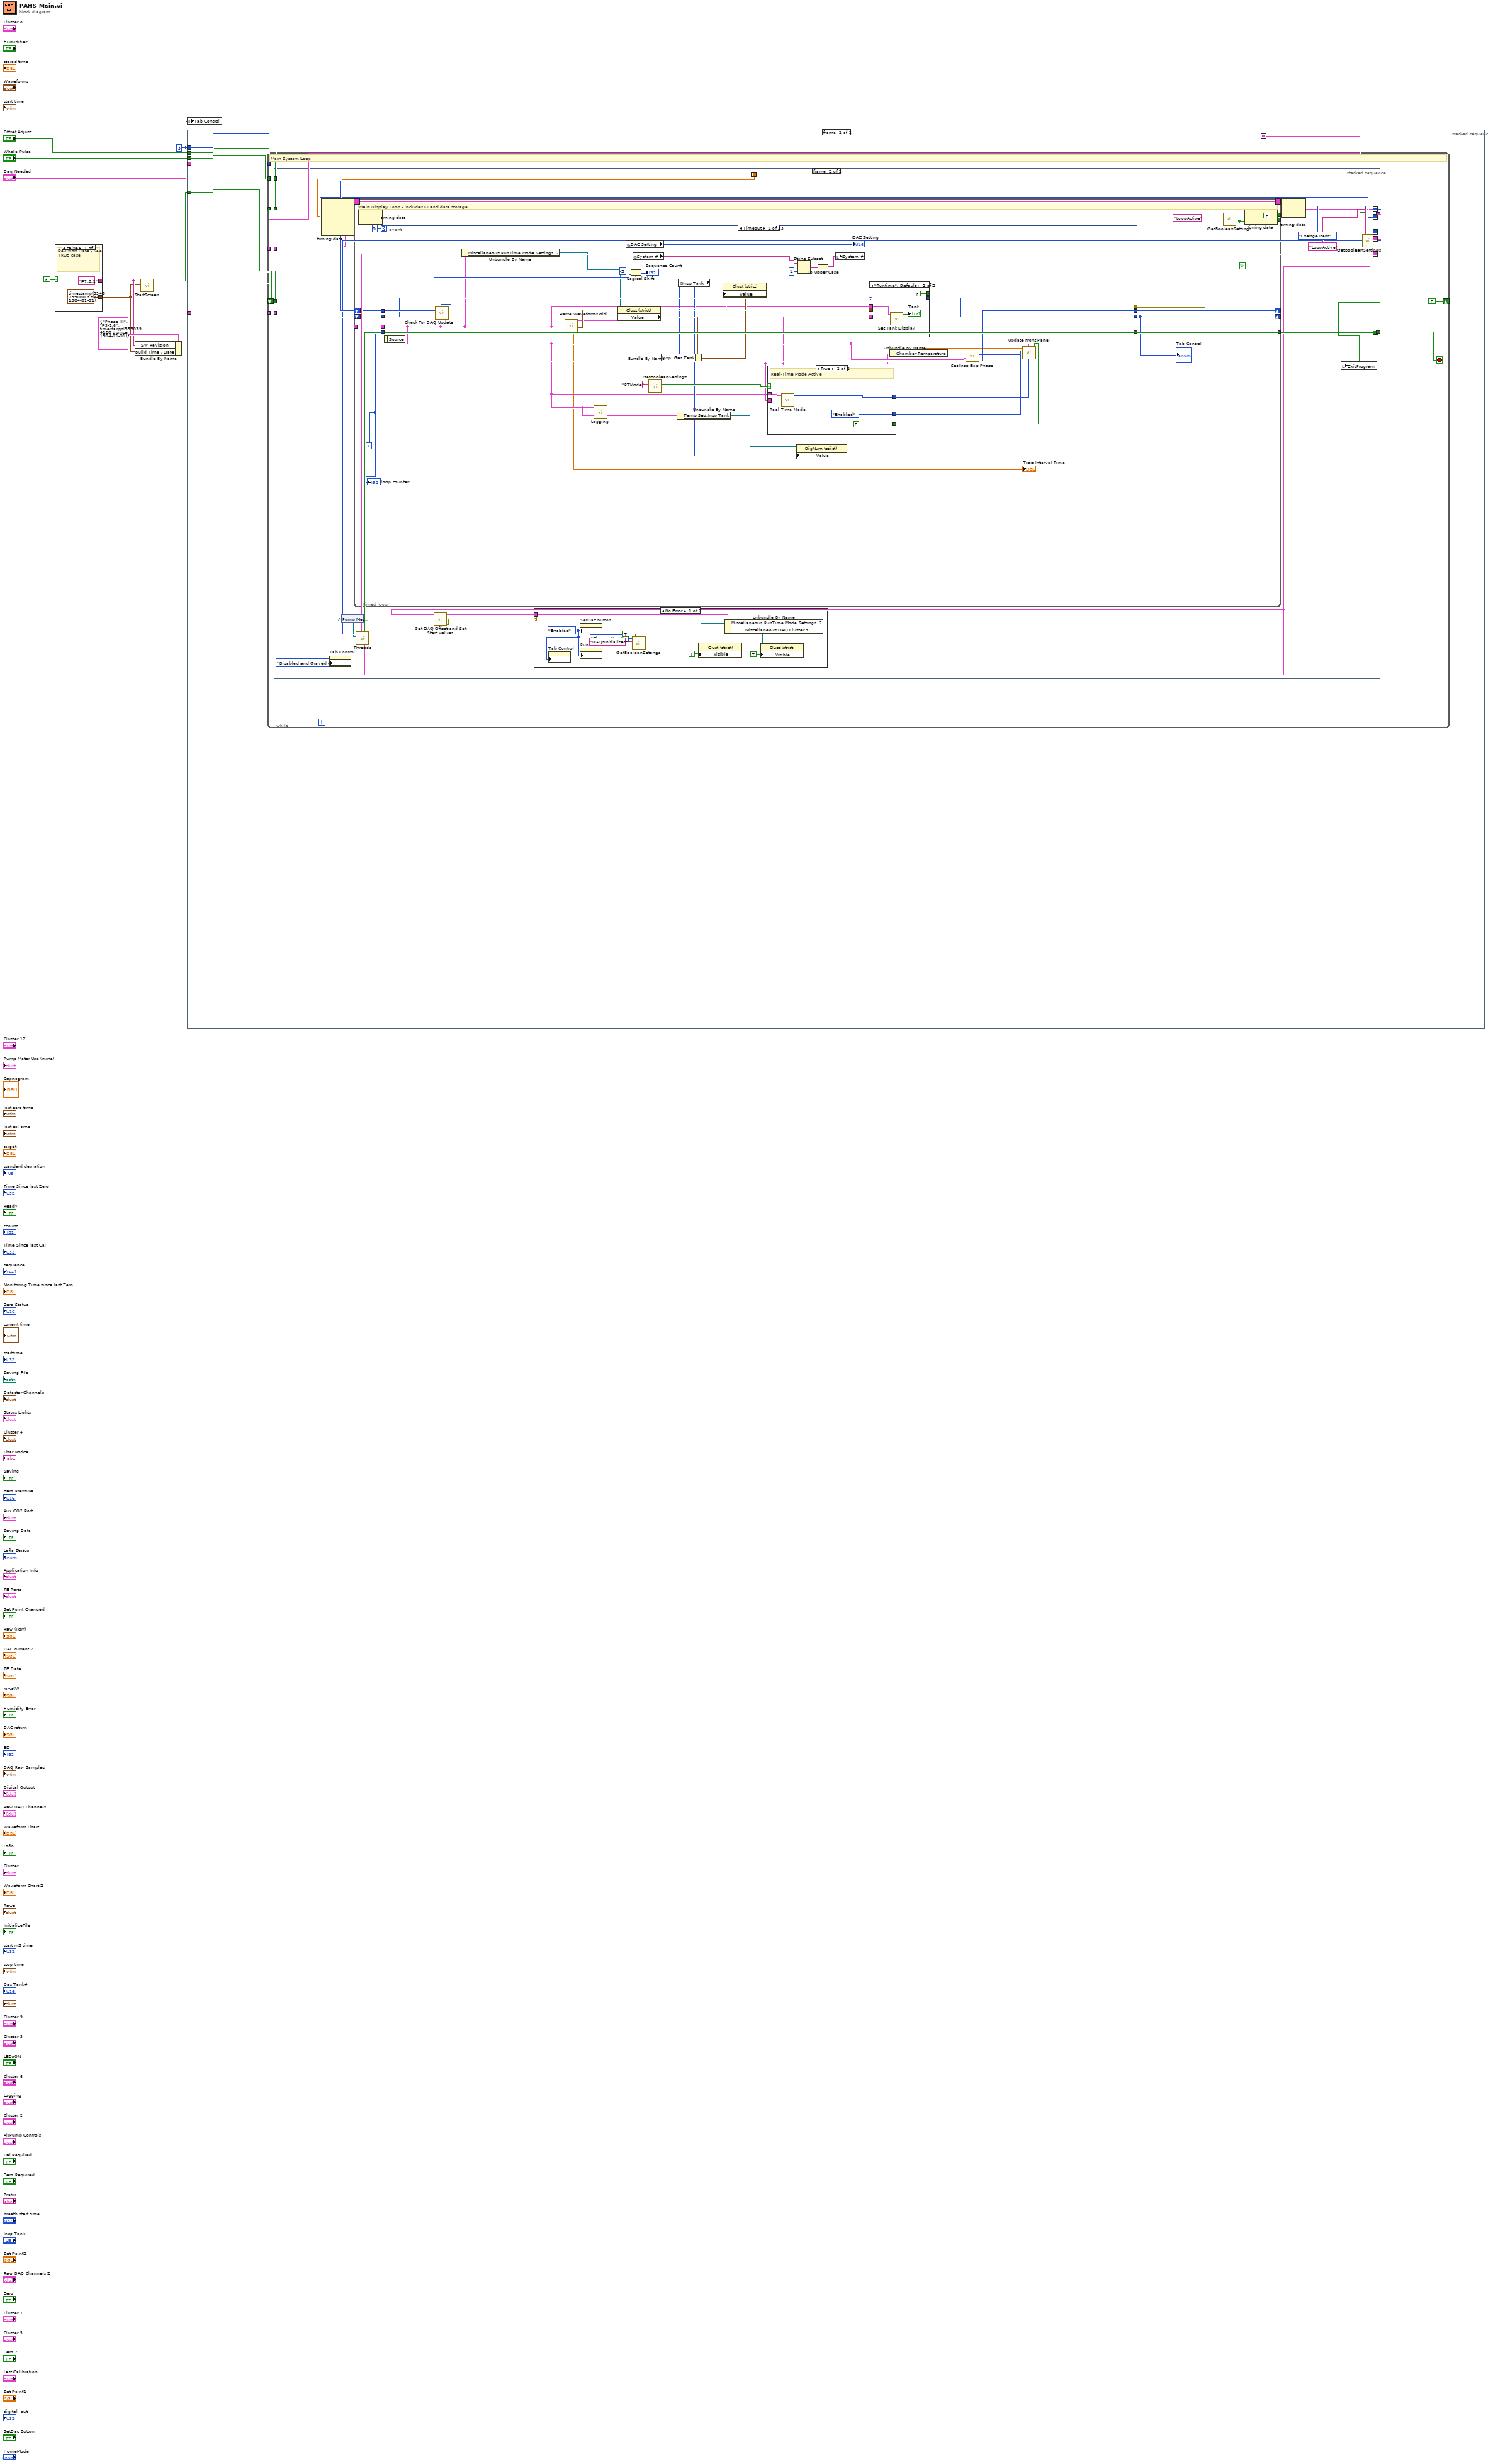
[diagram p0: block diagram]
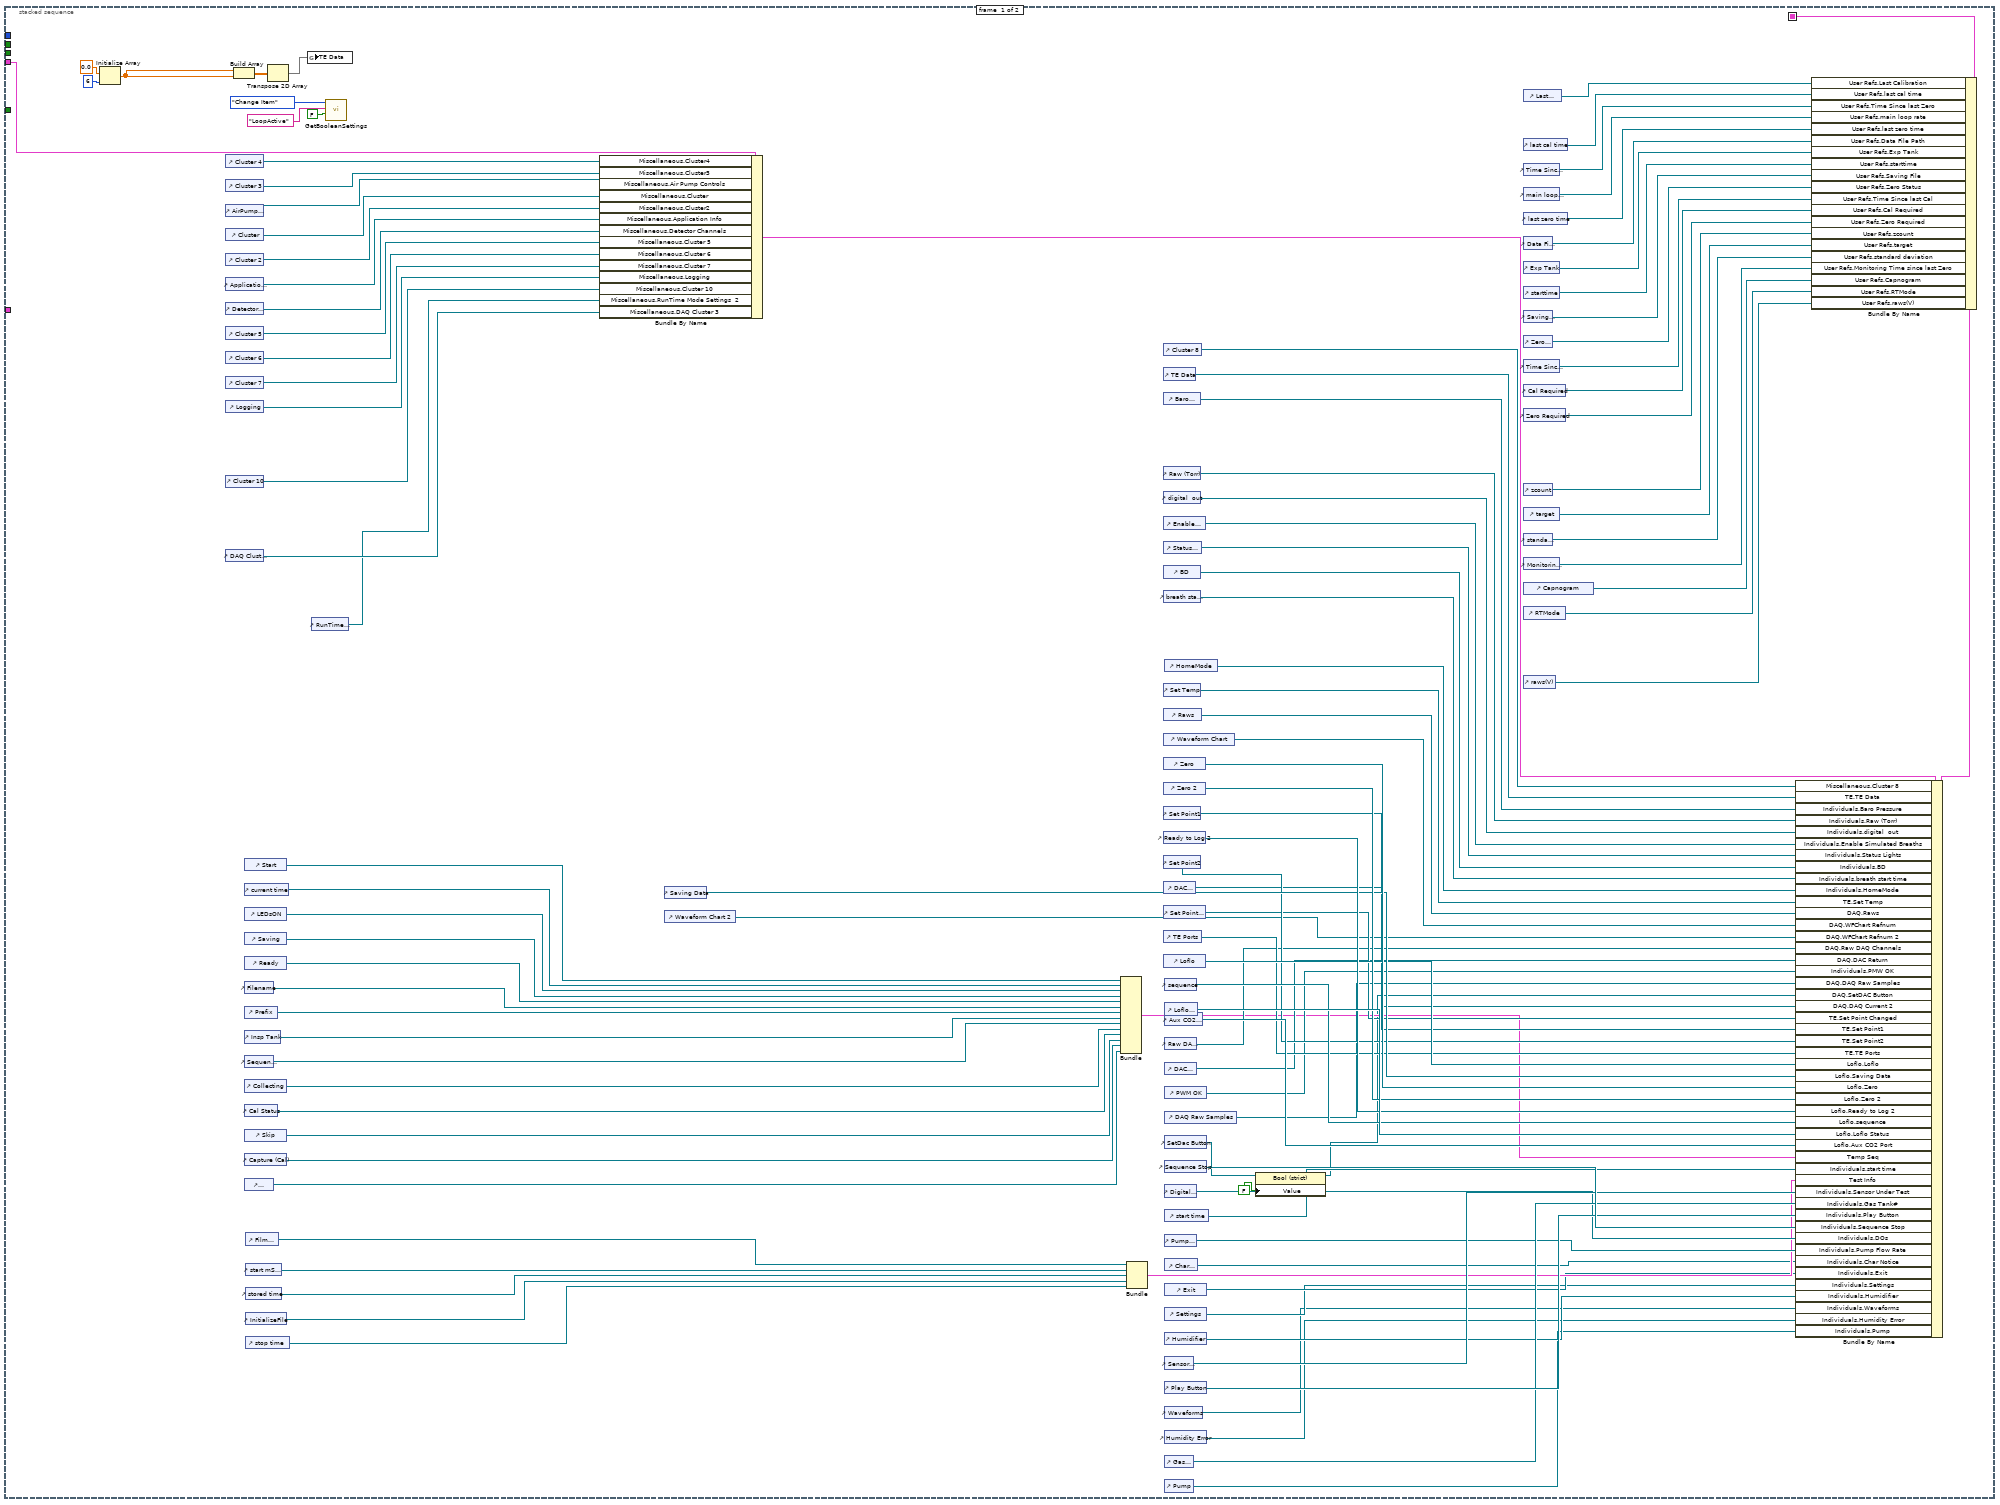
[diagram p2: hidden frame]
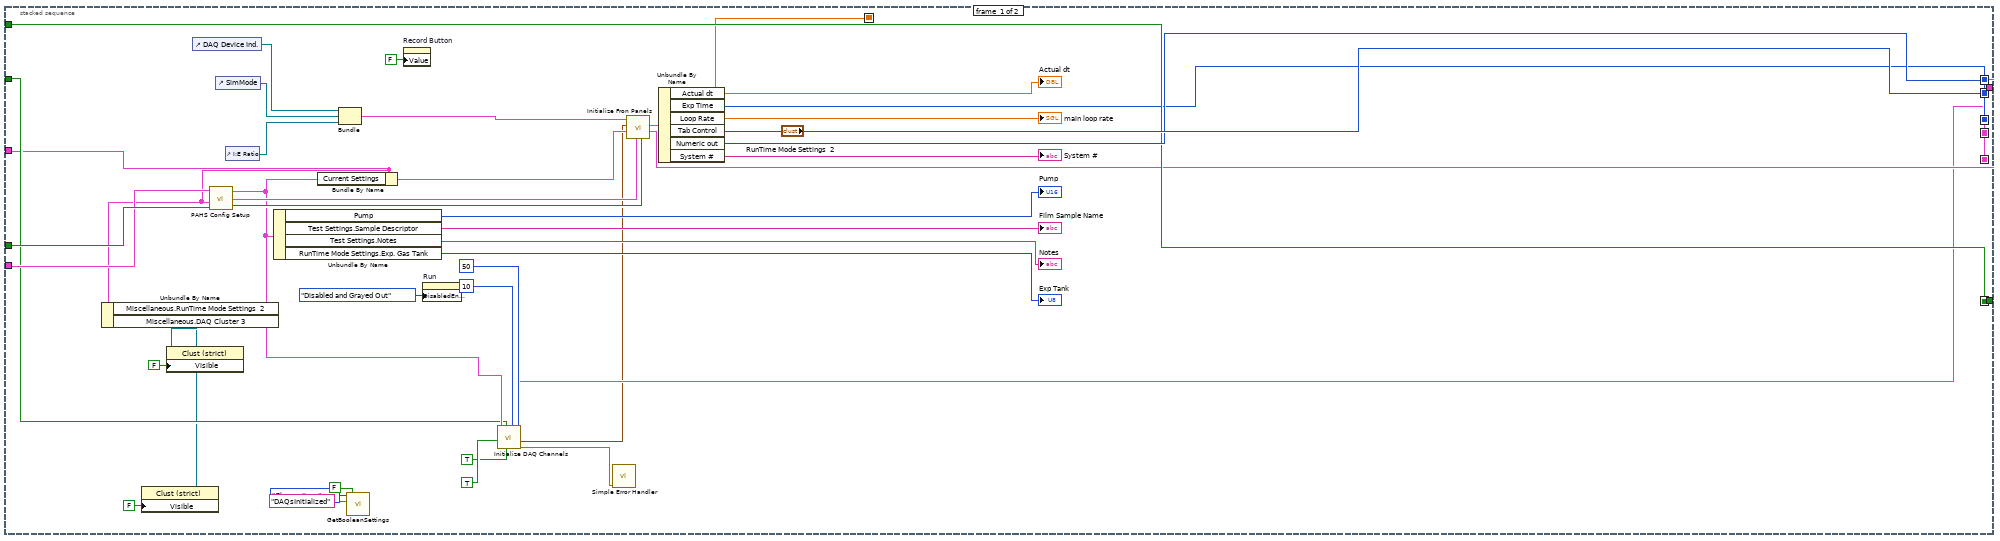
[diagram p3: hidden frame]
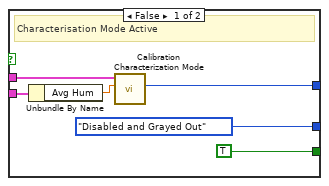
[diagram p4: hidden frame]
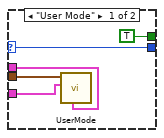
[diagram p5: hidden frame]
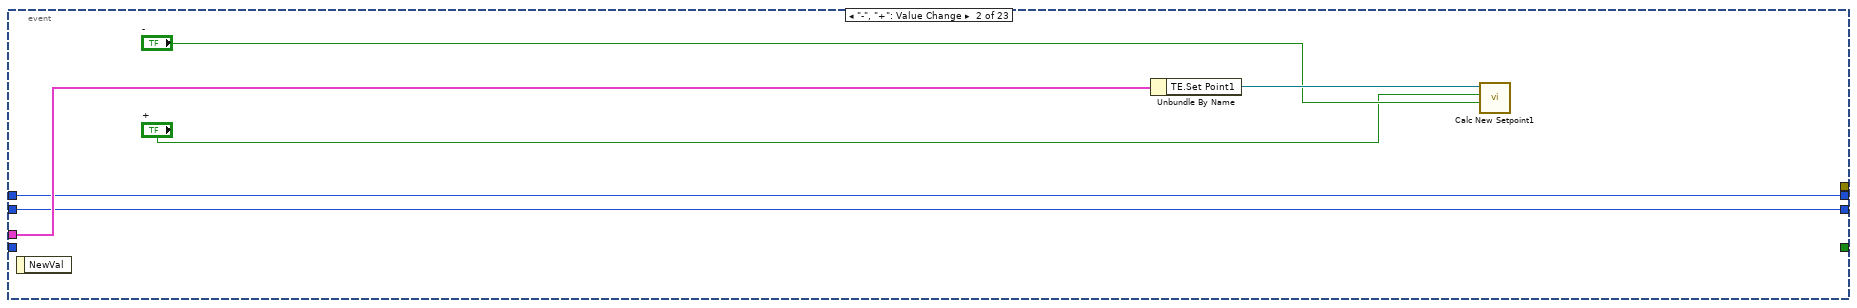
[diagram p6: hidden frame]
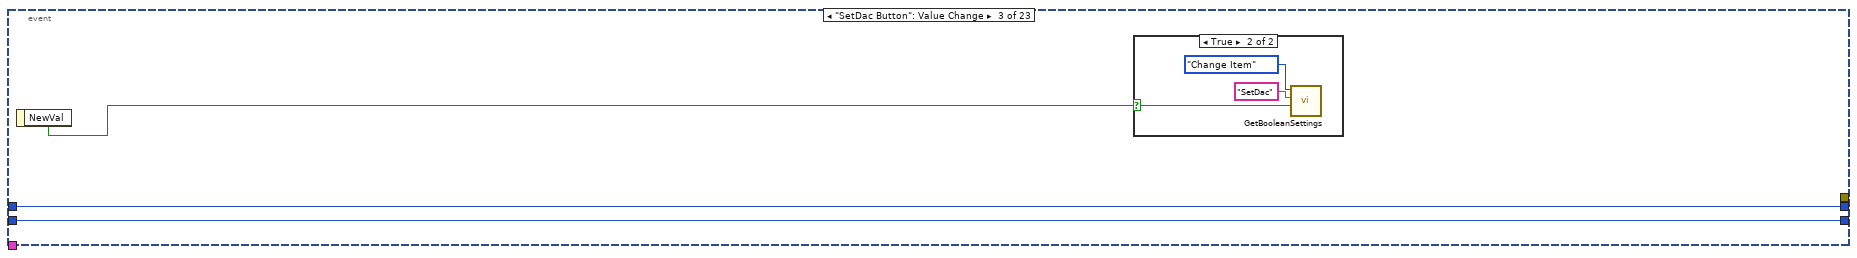
[diagram p7: hidden frame]
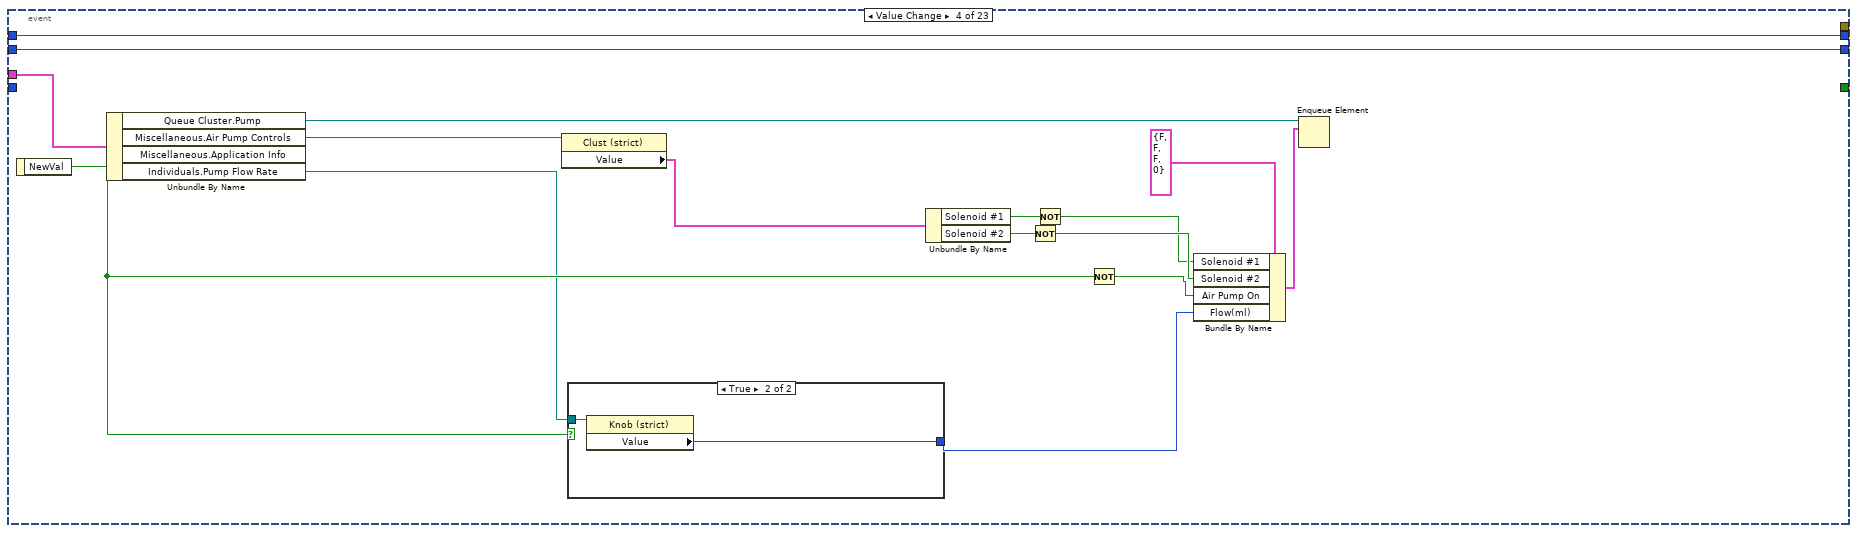
[diagram p9: hidden frame]
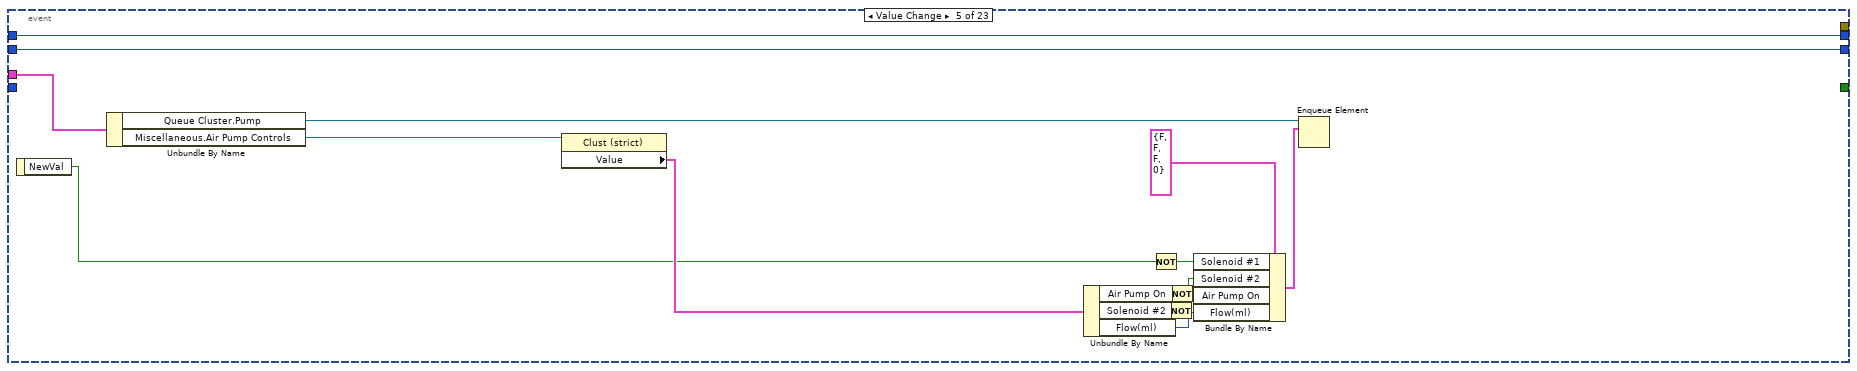
[diagram p11: hidden frame]
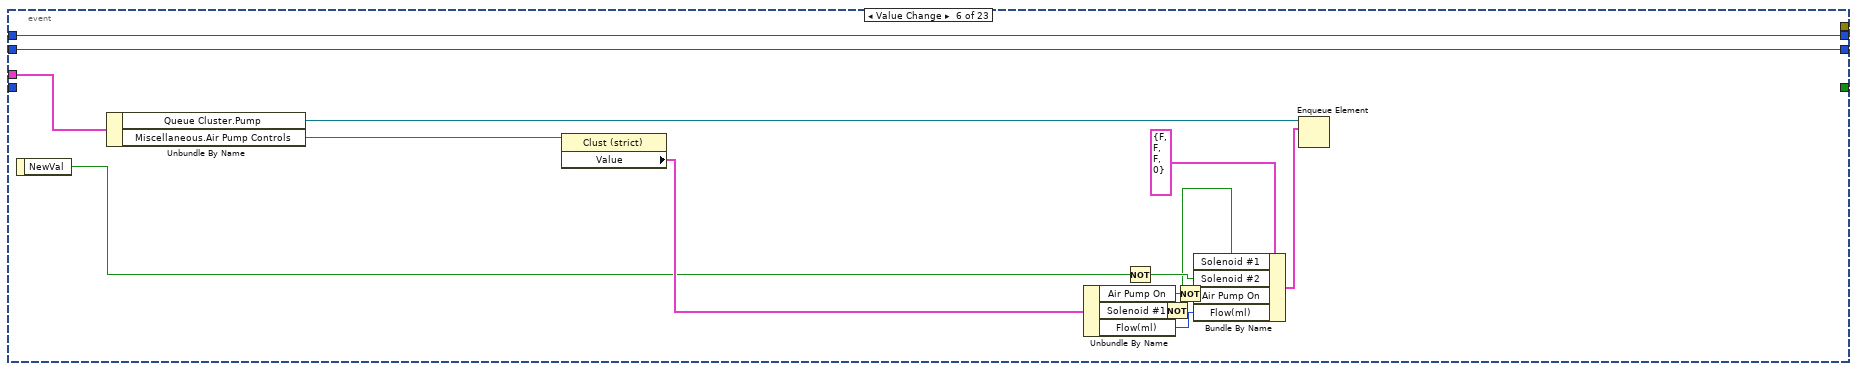
[diagram p12: hidden frame]
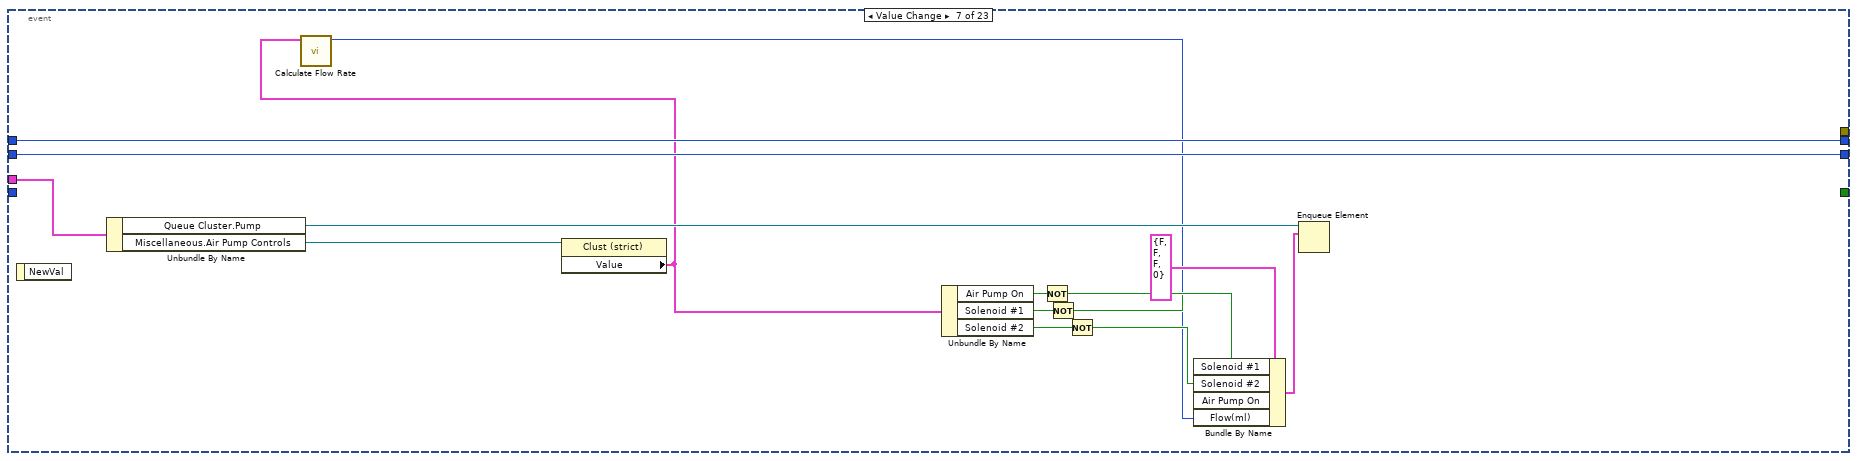
[diagram p13: hidden frame]
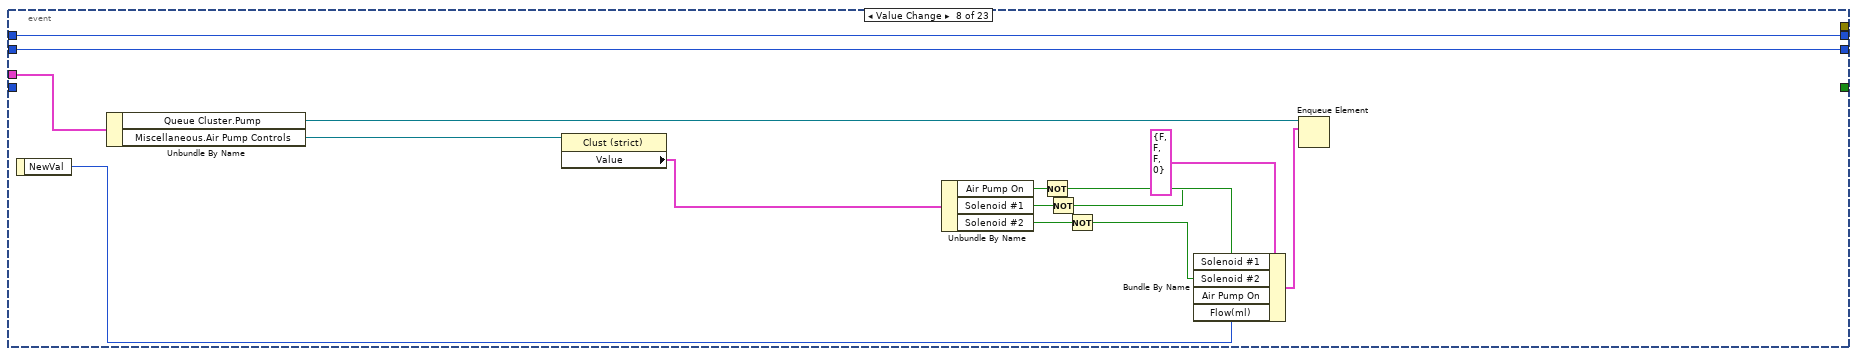
[diagram p14: hidden frame]
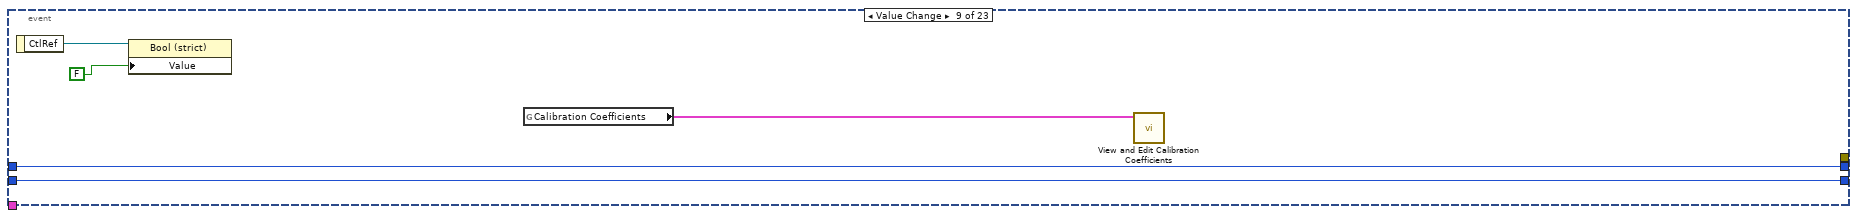
[diagram p15: hidden frame]
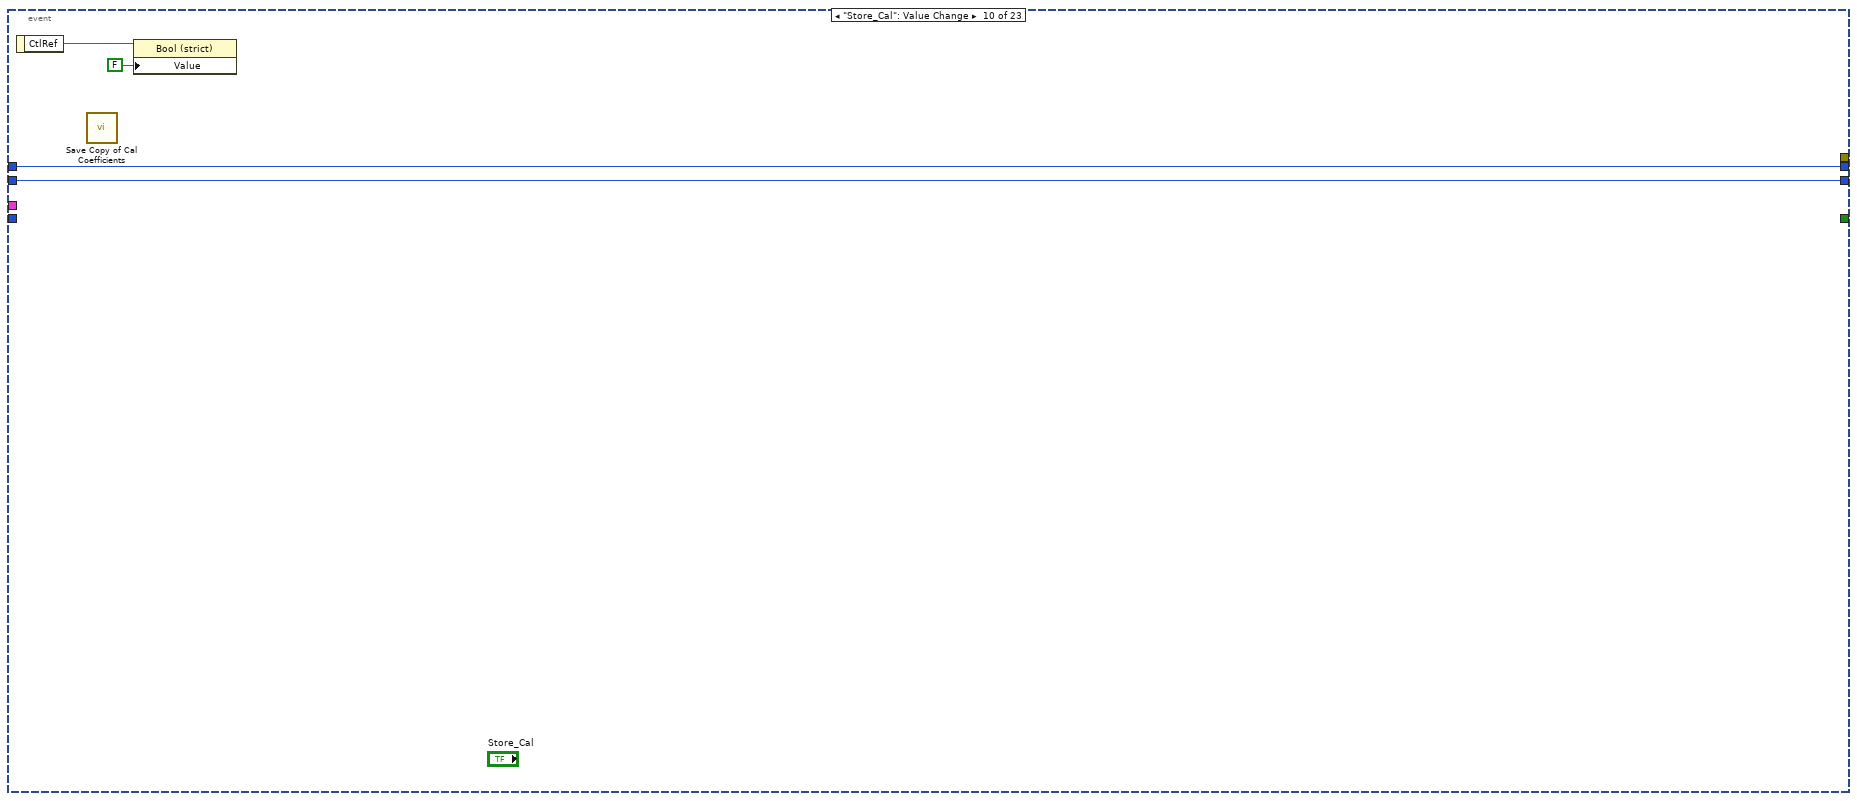
[diagram p16: hidden frame]
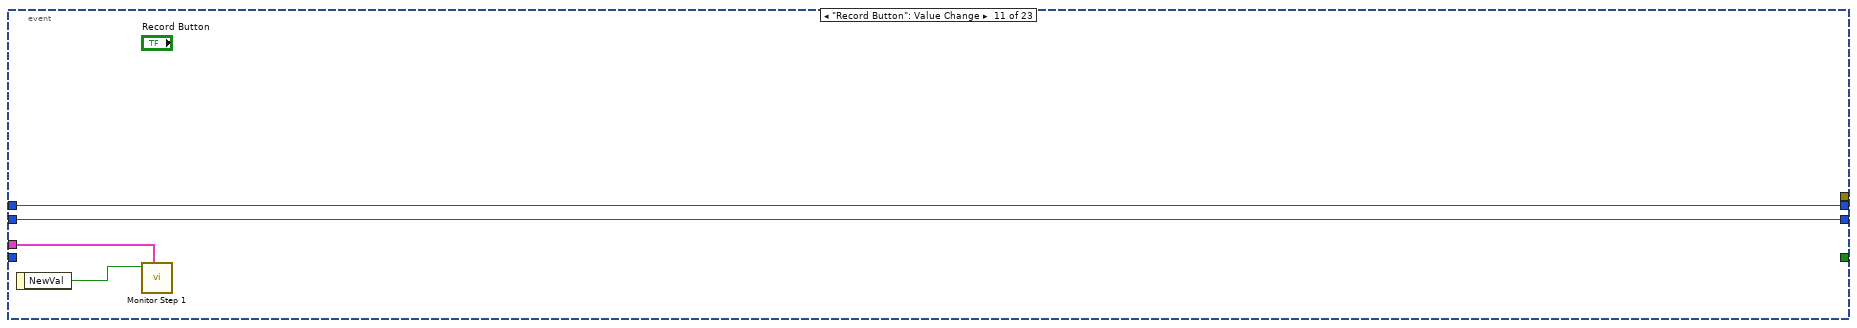
[diagram p17: hidden frame]
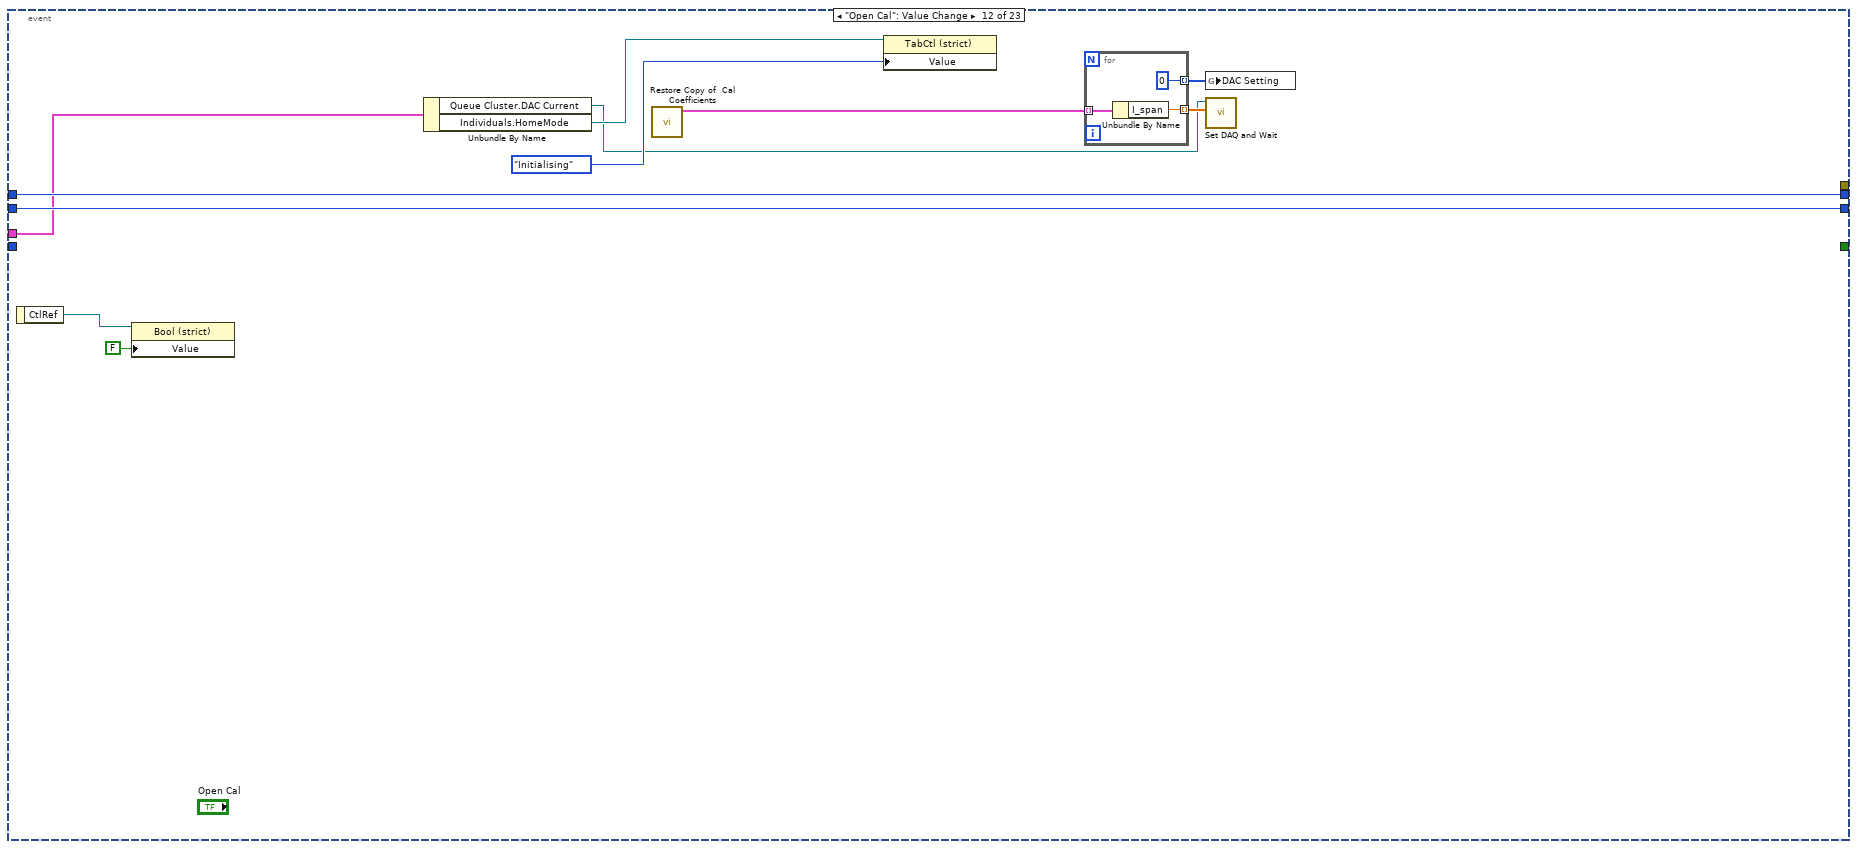
[diagram p18: hidden frame]
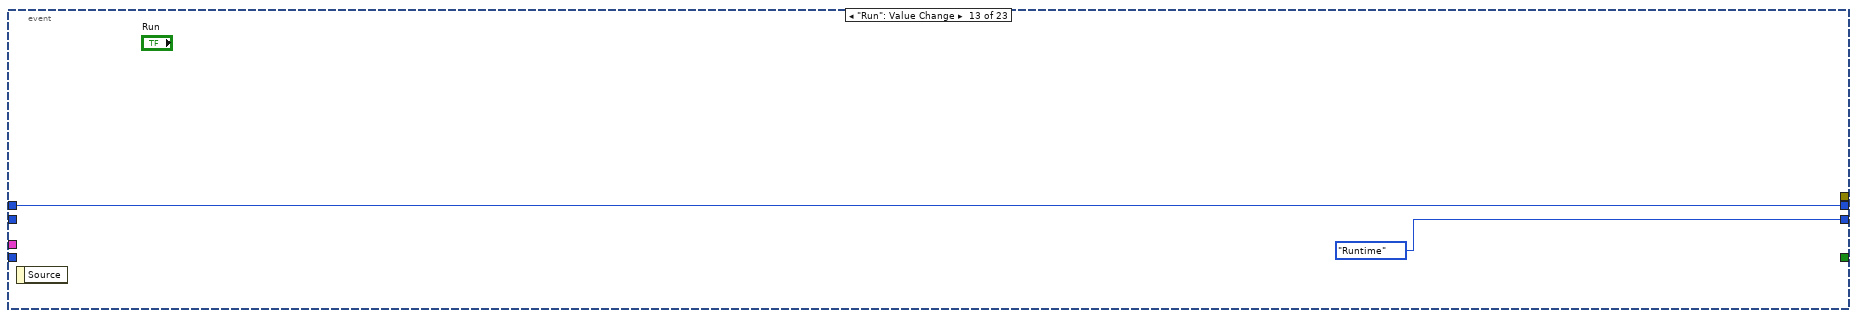
[diagram p19: hidden frame]
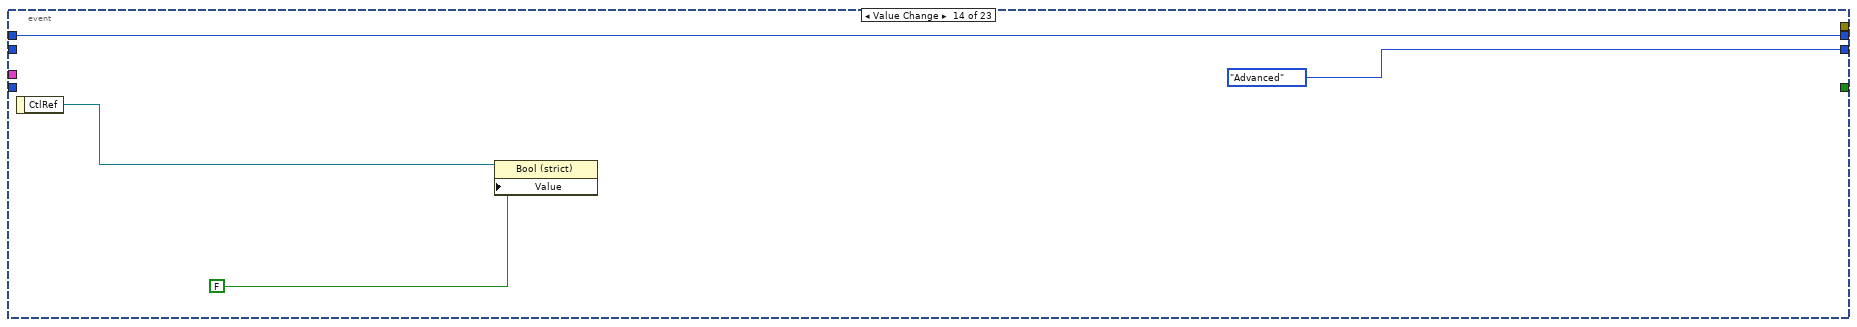
[diagram p20: hidden frame]
diagram:
  w10 = 3
  n1 = case shown="False" FALSE {
    tunnel: [timestamp(3548799000 s since 1904-01-01) ("Build Time / Date") w14] -> w2
    tunnel: ["P7.0.2" ("SW Revision") "X.X.X" ("SW Revision")] -> w3
    frame False {
      # "Revision Date - See TRUE case"
    }
    frame True {
      # "When True Sets New  Revision Time and Date - copy into constant in FALSE case"
      n2 = Get Date/Time In Seconds() -> (seconds since 1Jan1904=w14:timestamp)
    }
  }
  n3 = Bundle By Name(cluster=T39 {"SW Phase"="Phase III", "SW Revision"="P3-1.6", "Build Time / Date"=timestamp(3530394120 s since 1904-01-01)} ("Application Info"), "SW Revision"=w3, "Build Time / Date"=w2) -> (w1:T39)
  n4 = call "StartScreen.vi"("seconds since 1Jan1904"=w2, "SW Revision"=w3) -> ("T button?"=w8:bool)  [unwired: 9 in]
  n5 = local write "Tab Control"(w10) -> ()
  n6 = stacked-sequence {
    seq-local: [w109 _] -> [_ w133]
    tunnel: w10 -> [_ w135]
    tunnel: w8 -> [_ w134]
    tunnel: "Daq Needed" -> [w42 _]
    tunnel: "Whole Pulse" -> [_ w132]
    tunnel: "Offset Adjust" -> [_ w131]
    tunnel: w1 -> [_ w130]
    frame #0 {
      n7 = Initialize Array(0.0 ("element"), 6 ("dimension size")) -> (w56:dbl[])
      n8 = control-ref of="Cluster 4"() -> (w40:refnum<vi>)
      n9 = control-ref of="Cluster 3"() -> (w39:refnum<vi>)
      n10 = control-ref of="AirPump Controls"() -> (w38:refnum<vi>)
      n11 = control-ref of="Cluster"() -> (w37:refnum<vi>)
      n12 = control-ref of="Cluster 2"() -> (w36:refnum<vi>)
      n13 = control-ref of="Application Info"() -> (w35:refnum<vi>)
      n14 = control-ref of="Detector Channels"() -> (w34:refnum<vi>)
      n15 = control-ref of="Cluster 5"() -> (w33:refnum<vi>)
      n16 = control-ref of="Cluster 6"() -> (w32:refnum<vi>)
      n17 = control-ref of="Cluster 7"() -> (w31:refnum<vi>)
      n18 = control-ref of="Logging"() -> (w30:refnum<vi>)
      n19 = control-ref of="Cluster 10"() -> (w29:refnum<vi>)
      n20 = control-ref of="DAQ Cluster 3"() -> (w16:refnum<vi>)
      n21 = Build Array(w56, w56) -> (w57:dbl[][])
      n22 = control-ref of="Start"() -> (w60:refnum<vi>)
      n23 = control-ref of="current time"() -> (w61:refnum<vi>)
      n24 = control-ref of="LEDsON"() -> (w62:refnum<vi>)
      n25 = control-ref of="Saving"() -> (w63:refnum<vi>)
      n26 = control-ref of="Ready"() -> (w64:refnum<vi>)
      n27 = control-ref of="Filename"() -> (w65:refnum<vi>)
      n28 = control-ref of="Prefix"() -> (w66:refnum<vi>)
      n29 = control-ref of="Insp Tank"() -> (w67:refnum<vi>)
      n30 = control-ref of="Sequence Filename"() -> (w68:refnum<vi>)
      n31 = control-ref of="Collecting"() -> (w69:refnum<vi>)
      n32 = control-ref of="Cal Status"() -> (w70:refnum<vi>)
      n33 = control-ref of="Skip"() -> (w71:refnum<vi>)
      n34 = control-ref of="Capture (Cal)"() -> (w72:refnum<vi>)
      n35 = control-ref of="Characterisation Filename"() -> (w20:refnum<vi>)
      n36 = control-ref of="Film Sample Name"() -> (w48:refnum<vi>)
      n37 = control-ref of="start mS time"() -> (w47:refnum<vi>)
      n38 = control-ref of="stored time"() -> (w46:refnum<vi>)
      n39 = control-ref of="InitializeFile"() -> (w45:refnum<vi>)
      n40 = control-ref of="stop time"() -> (w44:refnum<vi>)
      n41 = Transpose 2D Array(2D array=w57) -> (transposed array=w58:dbl[][])
      n42 = global write "Globals.vi" "TE Data"(w58) -> ()
      n43 = control-ref of="RunTime Mode Settings  2"() -> (w15:refnum<vi>)
      n44 = call "GetBooleanSettings.vi"("Change Value"=FALSE, "Variable Name"="LoopActive", "Mode"=T40."Change Item") -> ()  [unwired: 1 in, 4 out]
      n45 = Bundle By Name(cluster=w42, "Miscellaneous.Cluster4"=w40, "Miscellaneous.Cluster3"=w39, "Miscellaneous.Air Pump Controls"=w38, "Miscellaneous.Cluster"=w37, "Miscellaneous.Cluster2"=w36, "Miscellaneous.Application Info"=w35, "Miscellaneous.Detector Channels"=w34, "Miscellaneous.Cluster 5"=w33, "Miscellaneous.Cluster 6"=w32, "Miscellaneous.Cluster 7"=w31, "Miscellaneous.Logging"=w30, "Miscellaneous.Cluster 10"=w29, "Miscellaneous.RunTime Mode Settings  2"=w15, "Miscellaneous.DAQ Cluster 3"=w16) -> (w41:T4)
      n46 = control-ref of="Saving Data"() -> (w91:refnum<vi>)
      n47 = control-ref of="Waveform Chart 2"() -> (w80:refnum<vi>)
      n48 = Bundle("Start"=w60, "current time"=w61, "LEDsON"=w62, "Saving"=w63, "Ready"=w64, "Filename"=w65, "Prefix"=w66, "Insp Tank"=w67, "Sequence Filename"=w68, "Collecting"=w69, "Cal Status"=w70, "Skip"=w71, "Capture (Cal)"=w72, "Characterisation Filename"=w20) -> (w59:T46)  [unwired: 1 in]
      n49 = Bundle("Film Sample Name"=w48, "start mS time"=w47, "stored time"=w46, "InitializeFile"=w45, "stop time"=w44) -> (w43:T47)  [unwired: 1 in]
      n50 = control-ref of="Cluster 8"() -> (w21:refnum<vi>)
      n51 = control-ref of="TE Data"() -> (w73:refnum<vi>)
      n52 = control-ref of="Baro Pressure"() -> (w75:refnum<vi>)
      n53 = control-ref of="Raw (Torr)"() -> (w76:refnum<vi>)
      n54 = control-ref of="digital  out"() -> (w77:refnum<vi>)
      n55 = control-ref of="Enable Simulated Breaths"() -> (w98:refnum<vi>)
      n56 = control-ref of="Status Lights"() -> (w100:refnum<vi>)
      n57 = control-ref of="BD"() -> (w101:refnum<vi>)
      n58 = control-ref of="breath start time"() -> (w102:refnum<vi>)
      n59 = control-ref of="Set Temp"() -> (w99:refnum<vi>)
      n60 = control-ref of="Raws"() -> (w78:refnum<vi>)
      n61 = control-ref of="Waveform Chart"() -> (w79:refnum<vi>)
      n62 = control-ref of="Zero"() -> (w92:refnum<vi>)
      n63 = control-ref of="Zero 2"() -> (w93:refnum<vi>)
      n64 = control-ref of="Set Point1"() -> (w87:refnum<vi>)
      n65 = control-ref of="Ready to Log 2"() -> (w94:refnum<vi>)
      n66 = control-ref of="Set Point2"() -> (w88:refnum<vi>)
      n67 = control-ref of="DAC current 2"() -> (w85:refnum<vi>)
      n68 = control-ref of="Set Point Changed"() -> (w86:refnum<vi>)
      n69 = control-ref of="TE Ports"() -> (w89:refnum<vi>)
      n70 = control-ref of="Loflo"() -> (w90:refnum<vi>)
      n71 = control-ref of="HomeMode"() -> (w103:refnum<vi>)
      n72 = control-ref of="sequence"() -> (w95:refnum<vi>)
      n73 = control-ref of="Loflo Status"() -> (w96:refnum<vi>)
      n74 = control-ref of="Aux CO2 Port"() -> (w97:refnum<vi>)
      n75 = control-ref of="Raw DAQ Channels"() -> (w81:refnum<vi>)
      n76 = control-ref of="DAC return"() -> (w82:refnum<vi>)
      n77 = control-ref of="PWM OK"() -> (w83:refnum<vi>)
      n78 = control-ref of="DAQ Raw Samples"() -> (w84:refnum<vi>)
      n79 = control-ref of="SetDac Button"() -> (w19:refnum<vi>)
      n80 = control-ref of="Sequence Stop"() -> (w108:refnum<vi>)
      n81 = control-ref of="Digital Output"() -> (w50:refnum<vi>)
      n82 = control-ref of="start time"() -> (w104:refnum<vi>)
      n83 = control-ref of="Pump Flow Rate"() -> (w49:refnum<vi>)
      n84 = control-ref of="Char Notice"() -> (w28:refnum<vi>)
      n85 = control-ref of="Exit"() -> (w27:refnum<vi>)
      n86 = control-ref of="Settings"() -> (w26:refnum<vi>)
      n87 = control-ref of="Humidifier"() -> (w25:refnum<vi>)
      n88 = control-ref of="Sensor Under Test"() -> (w105:refnum<vi>)
      n89 = control-ref of="Play Button"() -> (w107:refnum<vi>)
      n90 = control-ref of="Waveforms"() -> (w24:refnum<vi>)
      n91 = control-ref of="Humidity Error"() -> (w23:refnum<vi>)
      n92 = control-ref of="Gas Tank#"() -> (w106:refnum<vi>)
      n93 = control-ref of="Pump"() -> (w22:refnum<vi>)
      n94 = property class="Bool (strict)"(reference=w19, "Value"=FALSE) -> (reference out=w18:refnum<vi>)  [unwired: 1 in, 1 out]
      n95 = control-ref of="Last Calibration"() -> (w125:refnum<vi>)
      n96 = control-ref of="last cal time"() -> (w117:refnum<vi>)
      n97 = control-ref of="Time Since last Zero"() -> (w118:refnum<vi>)
      n98 = control-ref of="main loop rate"() -> (w119:refnum<vi>)
      n99 = control-ref of="last zero time"() -> (w120:refnum<vi>)
      n100 = control-ref of="Data File Path"() -> (w121:refnum<vi>)
      n101 = control-ref of="Exp Tank"() -> (w122:refnum<vi>)
      n102 = control-ref of="starttime"() -> (w123:refnum<vi>)
      n103 = control-ref of="Saving File"() -> (w124:refnum<vi>)
      n104 = control-ref of="Zero Status"() -> (w116:refnum<vi>)
      n105 = control-ref of="Time Since last Cal"() -> (w115:refnum<vi>)
      n106 = control-ref of="Cal Required"() -> (w114:refnum<vi>)
      n107 = control-ref of="Zero Required"() -> (w113:refnum<vi>)
      n108 = control-ref of="zcount"() -> (w112:refnum<vi>)
      n109 = control-ref of="target"() -> (w111:refnum<vi>)
      n110 = control-ref of="standard deviation"() -> (w110:refnum<vi>)
      n111 = control-ref of="Monitoring Time since last Zero"() -> (w126:refnum<vi>)
      n112 = control-ref of="Capnogram"() -> (w127:refnum<vi>)
      n113 = control-ref of="RTMode"() -> (w128:refnum<vi>)
      n114 = control-ref of="raws(V)"() -> (w129:refnum<vi>)
      n115 = Bundle By Name(cluster=w41, "Miscellaneous.Cluster 8"=w21, "TE.TE Data"=w73, "Individuals.Baro Pressure"=w75, "Individuals.Raw (Torr)"=w76, "Individuals.digital  out"=w77, "Individuals.Enable Simulated Breaths"=w98, "Individuals.Status Lights"=w100, "Individuals.BD"=w101, "Individuals.breath start time"=w102, "Individuals.HomeMode"=w103, "TE.Set Temp"=w99, "DAQ.Raws"=w78, "DAQ.WFChart Refnum"=w79, "DAQ.WFChart Refnum 2"=w80, "DAQ.Raw DAQ Channels"=w81, "DAQ.DAC Return"=w82, "Individuals.PMW OK"=w83, "DAQ.DAQ Raw Samples"=w84, "DAQ.SetDAC Button"=w18, "DAQ.DAQ Current 2"=w85, "TE.Set Point Changed"=w86, "TE.Set Point1"=w87, "TE.Set Point2"=w88, "TE.TE Ports"=w89, "Loflo.Loflo"=w90, "Loflo.Saving Data"=w91, "Loflo.Zero"=w92, "Loflo.Zero 2"=w93, "Loflo.Ready to Log 2"=w94, "Loflo.sequence"=w95, "Loflo.Loflo Status"=w96, "Loflo.Aux CO2 Port"=w97, "Temp Seq"=w59, "Individuals.start time"=w104, "Test Info"=w43, "Individuals.Sensor Under Test"=w105, "Individuals.Gas Tank#"=w106, "Individuals.Play Button"=w107, "Individuals.Sequence Stop"=w108, "Individuals.DOs"=w50, "Individuals.Pump Flow Rate"=w49, "Individuals.Char Notice"=w28, "Individuals.Exit"=w27, "Individuals.Settings"=w26, "Individuals.Humidifier"=w25, "Individuals.Waveforms"=w24, "Individuals.Humidity Error"=w23, "Individuals.Pump"=w22) -> (w74:T4)
      n116 = Bundle By Name(cluster=w74, "User Refs.Last Calibration"=w125, "User Refs.last cal time"=w117, "User Refs.Time Since last Zero"=w118, "User Refs.main loop rate"=w119, "User Refs.last zero time"=w120, "User Refs.Data File Path"=w121, "User Refs.Exp Tank"=w122, "User Refs.starttime"=w123, "User Refs.Saving File"=w124, "User Refs.Zero Status"=w116, "User Refs.Time Since last Cal"=w115, "User Refs.Cal Required"=w114, "User Refs.Zero Required"=w113, "User Refs.zcount"=w112, "User Refs.target"=w111, "User Refs.standard deviation"=w110, "User Refs.Monitoring Time since last Zero"=w126, "User Refs.Capnogram"=w127, "User Refs.RTMode"=w128, "User Refs.raws(V)"=w129) -> (w109:T4)
    }
    frame #1 {
      n117 = while {
        shift-right: [FALSE ("T button?")] -> _
        shift-left: w134 -> [w142]
        tunnel: w135 -> [_]
        tunnel: w133 -> [w141]
        tunnel: w132 -> [w140]
        tunnel: w131 -> [w139]
        tunnel: w130 -> [w138]
        stop <- w137 stop-if-true
        # "Main System Loop"
        n118 = stacked-sequence {
          seq-local: [w170 _] -> [_ w193]
          seq-local: [w171 _] -> [_ w198]
          seq-local: [w165 _] -> [_ w199]
          seq-local: [w164 _] -> [_ w184]
          seq-local: [w168 _] -> [_ w194]
          seq-local: [w155 _] -> [_ w191]
          seq-local: [w151 _] -> [_ w186]
          tunnel: w142 -> [w183 _]
          tunnel: w141 -> [w147 _]
          tunnel: w140 -> [w156 _]
          tunnel: w139 -> [w168 _]
          tunnel: w138 -> [w163 _]
          tunnel: [_ w184] -> _
          tunnel: [_ w190] -> w137
          frame #0 {
            n119 = Unbundle By Name(w147) -> ("Miscellaneous.RunTime Mode Settings  2"=w143:refnum<vi>, "Miscellaneous.DAQ Cluster 3"=w146:refnum<vi>)
            n120 = property class="Clust (strict)"(reference=w143, "Visible"=FALSE) -> ()  [unwired: 1 in, 2 out]
            n121 = property class="Clust (strict)"(reference=w146, "Visible"=FALSE) -> ()  [unwired: 1 in, 2 out]
            n122 = control-ref of="DAQ Device Ind."() -> (w178:refnum<vi>)
            n123 = call "PAHS Config Setup.vi"("AutoExit"=w183, "Refs"=w147, "Application Info"=w163) -> ("InUserMode"=w173:bool, "Output Parameters"=w172:T48, "Current Settings"=w157:T5)  [unwired: 1 in]
            n124 = control-ref of="SimMode"() -> (w177:refnum<vi>)
            n125 = control-ref of="I:E Ratio"() -> (w167:refnum<vi>)
            n126 = Unbundle By Name(w157) -> ("Pump"=→"Pump":u16, "Test Settings.Sample Descriptor"=→"Film Sample Name":string, "Test Settings.Notes"=→"Notes":string, "RunTime Mode Settings.Exp. Gas Tank"=→"Exp Tank":u16)
            n127 = Bundle By Name(cluster=w147, "Current Settings"=w157) -> (w166:T4)
            n128 = Bundle("DAQ Device Ind."=w178, "SimMode"=w177, "I:E Ratio"=w167) -> (w174:T49)  [unwired: 1 in]
            n129 = call "GetBooleanSettings.vi"("Change Value"=FALSE, "Variable Name"="DAQsInitialized", "Mode"=T40."Change Item") -> ()  [unwired: 1 in, 4 out]
            n130 = property on="Record Button" class="Bool (strict)"("Value"=FALSE ("Record Button")) -> ()  [unwired: 2 in, 2 out]
            n131 = property on="Run" class="Bool"("DisabledEnum"=T41."Disabled and Grayed Out" ("Disabled")) -> ()  [unwired: 2 in, 2 out]
            n132 = call "Initialize DAQ Channels.vi"("Air Pump PWM%"=u16 50, "Number of Aux Analog Channels"=u8 10, "Invert Signal"=TRUE, "Fast Sample"=w156, "Invert Digital Outputs"=TRUE, "Current Settings"=w157) -> ("error out"=w158:errorcluster, "SampleRateData"=w154:T50, "DAQTasks"=w155:T51)  [unwired: 2 in]
            n133 = call <vilib>:"Simple Error Handler.vi"("error in (no error)"=w158) -> ()  [unwired: 4 in, 5 out]
            n134 = call "Initialize Fron Panels.vi"("InUserMode"=w173, "Output Parameters"=w172, "Daq Needed"=w166, "SampleRateData"=w154, "output cluster"=w174) -> ("output cluster 2"=w164:T4, "output cluster 3"=w176:T52)  [unwired: 5 in]
            n135 = Unbundle By Name(w176) -> ("Actual dt"=→"Actual dt":dbl, "Exp Time"=w165:u32, "Loop Rate"=w151:dbl, "Tab Control"=w171:T13, "Numeric out"=w170:u32, "System #"=→"System #":string)
            "main loop rate" <- w151
          }
          frame #1 {
            n136 = node-c288(w186) -> (w188:T42)  [unwired: 3 in]
            n137 = property on="Tab Control" class="TabCtl (strict)"("DisabledEnum"=T41."Disabled and Grayed Out" ("Disabled")) -> ()  [unwired: 2 in, 2 out]
            n138 = control-ref of="Pump Meter Use (mins)"() -> (w192:refnum<vi>)
            n139 = timed-loop {
              tunnel: [w210] -> w190
              shift-right: [w204] -> _
              shift-left: w198 -> [w207]
              shift-right: [w211] -> _
              shift-left: w199 -> [w208]
              tunnel: [w205] -> w195
              tunnel: [FALSE ("LEDsON")] -> _
              tunnel: w184 -> [w200]
              timing: w188 -> [_]
              timing-out: [_] -> w187
              i -> [w202]
              stop <- w205 continue-if-true
              # "Main Display Loop - includes UI and data storage"
              n140 = node-c288() -> ()  [unwired: 1 in, 1 out]
              n141 = event shown="[0] Timeout" {
                selector: _ -> [_ _ _ _ _ _ _ _ _ _ _ _ _ _ _ _ _ _ _ _ _ _ _]
                dyn-events: _ -> [_ _ _ _ _ _ _ _ _ _ _ _ _ _ _ _ _ _ _ _ _ _ _]
                timeout: 0 -> [_ _ _ _ _ _ _ _ _ _ _ _ _ _ _ _ _ _ _ _ _ _ _]
                tunnel: [w242 w262 w269 w288 w305 w320 w335 w350 w355 w359 w363 w374 w380 w384 w391 w402 w410 w430 w453 w462 w474 w489 _] -> w211
                tunnel: [_ _ _ _ _ _ _ _ _ _ _ _ _ _ _ FALSE _ _ w442 w456 _ _ _] -> w210
                tunnel: w202 -> [w241 _ _ _ _ _ _ _ _ _ _ _ _ _ _ _ _ _ _ _ _ _ _]
                tunnel: [w240 w263 w270 w289 w306 w321 w336 w351 w356 w360 w364 w375 enum32{"User Mode", "Runtime", "Advanced"}."Runtime" ("Tab Control") enum32{"User Mode", "Runtime", "Advanced"}."Advanced" ("Tab Control") w387 w401 w409 w429 w452 w461 w473 w488 _] -> w204
                tunnel: w208 -> [w238 w262 w269 w288 w305 w320 w335 w350 w355 w359 w363 w374 w380 w384 w391 w402 w410 w430 w453 w462 w474 w489 _]
                tunnel: w207 -> [w236 w263 w270 w289 w306 w321 w336 w351 w356 w360 w364 w375 _ _ w387 w401 w409 w429 w452 w461 w473 w488 _]
                tunnel: w200 -> [w217 w267 _ w287 w304 w319 w334 w349 _ _ w361 w368 _ _ w385 w393 w408 w426 w443 w457 w475 w496 _]
                tunnel: [_ _ _ _ _ _ _ _ _ _ _ _ _ _ _ w400 _ _ w448 _ _ _ _] -> w203
                event Timeout {
                  n142 = event-data() -> ()  [unwired: 1 in, 1 out]
                  n143 = call "Check For DAQ Update.vi"("output cluster in"=w217, "Numeric"=w241) -> ()  [unwired: 10 in]
                  n144 = Unbundle By Name(w217) -> ("Miscellaneous.RunTime Mode Settings  2"=w216:refnum<vi>)
                  n145 = call "Parse Waveforms old.vi"("Daq Needed"=w217) -> ("Processed Variables"=w228:T12, "output cluster"=w214:T53, "Ticks Interval Time"=→"Ticks Interval Time":dbl)  [unwired: 5 in, 3 out]
                  n146 = call "Logging.vi"("output cluster in"=w217) -> ()  [unwired: 11 in]
                  n147 = property class="Clust (strict)"(reference=w216) -> (reference out=w221:refnum<vi>, "Value"=w220:T1)  [unwired: 1 in, 1 out]
                  n148 = global read "Globals.vi" "DAC Setting"() -> (→"DAC Setting":u16[])
                  n149 = Logical Shift(y=i16 -3, x=w238) -> (x << y=→"Sequence Count":u32)
                  n150 = global read "Globals.vi" "System #"() -> (w224:string)
                  n151 = call "GetBooleanSettings.vi"("Variable Name"="RTMode") -> ("Set Value"=w230:bool)  [unwired: 3 in, 3 out]
                  n152 = Unbundle By Name(w217) -> ("Temp Seq.Insp Tank"=w222:refnum<vi>)
                  n153 = global read "Globals.vi" "Insp Tank"() -> (w218:u16)
                  n154 = Bundle By Name(cluster=w220, "Insp. Gas Tank"=w218) -> (w219:T1)
                  n155 = property class="Clust (strict)"(reference=w221, "Value"=w219) -> ()  [unwired: 1 in, 2 out]
                  n156 = case shown="True" w230 {
                    tunnel: [T41."Disabled and Grayed Out" ("Disabled") T41."Enabled" ("Disabled")] -> w233
                    tunnel: [w248 w249] -> w235
                    tunnel: [TRUE FALSE] -> w229
                    tunnel: w217 -> [w245 w250]
                    tunnel: w214 -> [w244 _]
                    frame False {
                      # "Characterisation Mode Active"
                      n157 = Unbundle By Name(w244) -> ("Avg Hum"=w243:dbl)
                      n158 = call "Calibration Characterization Mode.vi"("Avg Hum"=w243, "Daq Needed"=w245) -> ("Disabled out"=w248:T41)  [unwired: 9 in]
                    }
                    frame True {
                      # "Real-Time Mode Active"
                      n159 = call "Real Time Mode.vi"("Daq Needed"=w250) -> ("Enabled"=w249:T41)  [unwired: 10 in]
                    }
                  }
                  n160 = property class="DigNum (strict)"(reference=w222, "Value"=w218) -> ()  [unwired: 1 in, 2 out]
                  n161 = String Subset(string=w224, length (rest)=1 ("length (rest)")) -> (substring=w225:string)  [unwired: 1 in]
                  n162 = To Upper Case(1:w225) -> (0:w223:string)
                  n163 = local write "System #"(w223) -> ()
                  n164 = case shown="\"Runtime\", Default" w236 {
                    selector: w236 -> [w257 w261]
                    tunnel: [w257 w261] -> w240
                    tunnel: [TRUE FALSE] -> _
                    tunnel: w228 -> [w255 _]
                    tunnel: w214 -> [w254 _]
                    tunnel: w217 -> [w253 w258]
                    frame "User Mode" {
                      n165 = call "UserMode.vi"("DAQ needed"=w253, "output cluster 2"=w254, "Processed Variables"=w255) -> ()  [unwired: 9 in]
                    }
                    frame "Runtime", Default {
                      n166 = call "Set Tank Display.vi"("output cluster 2"=w258) -> ("Boolean array"=→"Tank":bool[])  [unwired: 9 in, 1 out]
                    }
                  }
                  n167 = Unbundle By Name(w214) -> ("Chamber Temperature"=w227:dbl)
                  n168 = call "Set Insp-Exp Phase.vi"("counter in"=w238, "Daq Needed 2"=w217) -> ("counter out"=w242:u32, "GasTankOut"=w232:u8)  [unwired: 8 in]
                  n169 = call "Update Front Panel.vi"("Visible"=w229, "Disabled"=w235, "daq needed"=w217, "Set Value"=w232, "Disabled 2"=w233, "output cluster.Chamber Temperature"=w227) -> ()  [unwired: 6 in]
                }
                event "-", "+": Value Change {
                  n170 = event-data() -> ()  [unwired: 1 in, 1 out]
                  n171 = Unbundle By Name(w267) -> ("TE.Set Point1"=w266:refnum<vi>)
                  n172 = call "Calc New Setpoint1.vi"("-"="-", "+"="+", "Digital in"=w266) -> ()  [unwired: 9 in]
                }
                event "SetDac Button": Value Change {
                  n173 = event-data() -> ("NewVal"=w268:bool)  [unwired: 1 in]
                  n174 = case shown="True" w268 {
                    selector: w268 -> [_ w272]
                    frame False {
                    }
                    frame True {
                      n175 = call "GetBooleanSettings.vi"("Change Value"=w272, "Variable Name"="SetDac", "Mode"=T40."Change Item") -> ()  [unwired: 1 in, 4 out]
                    }
                  }
                }
                event Value Change {
                  n176 = event-data() -> ("NewVal"=w279:bool)  [unwired: 1 in]
                  n177 = Unbundle By Name(w287) -> ("Queue Cluster.Pump"=w285:refnum<queue>, "Miscellaneous.Air Pump Controls"=w286:refnum<vi>, "Individuals.Pump Flow Rate"=w278:refnum<vi>)  [unwired: 1 out]
                  n178 = property class="Clust (strict)"(reference=w286) -> ("Value"=w283:T35)  [unwired: 1 in, 2 out]
                  n179 = case shown="True" w279 {
                    tunnel: w278 -> [_ w291]
                    tunnel: [_ w290] -> w277
                    frame False {
                    }
                    frame True {
                      n180 = property class="Knob (strict)"(reference=w291) -> ("Value"=w290:u16)  [unwired: 1 in, 2 out]
                    }
                  }
                  n181 = Unbundle By Name(w283) -> ("Solenoid #1"=w282:bool, "Solenoid #2"=w281:bool)
                  n182 = Not(x=w281) -> (.not. x?=w275:bool)
                  n183 = Not(x=w282) -> (.not. x?=w274:bool)
                  n184 = Not(x=w279) -> (.not. x?=w276:bool)
                  n185 = Bundle By Name(cluster=T45 {"Solenoid #1"=FALSE, "Solenoid #2"=FALSE, "Air Pump On"=FALSE, "Flow(ml)"=0} ("element"), "Solenoid #1"=w274, "Solenoid #2"=w275, "Air Pump On"=w276, "Flow(ml)"=w277) -> (w280:T45)
                  n186 = Enqueue Element(queue=w285, element=w280) -> ()  [unwired: 2 in, 3 out]
                }
                event Value Change {
                  n187 = event-data() -> ("NewVal"=w296:bool)  [unwired: 1 in]
                  n188 = Unbundle By Name(w304) -> ("Queue Cluster.Pump"=w302:refnum<queue>, "Miscellaneous.Air Pump Controls"=w303:refnum<vi>)
                  n189 = property class="Clust (strict)"(reference=w303) -> ("Value"=w300:T35)  [unwired: 1 in, 2 out]
                  n190 = Unbundle By Name(w300) -> ("Air Pump On"=w295:bool, "Solenoid #2"=w299:bool, "Flow(ml)"=w298:u16)
                  n191 = Not(x=w296) -> (.not. x?=w294:bool)
                  n192 = Not(x=w299) -> (.not. x?=w292:bool)
                  n193 = Not(x=w295) -> (.not. x?=w293:bool)
                  n194 = Bundle By Name(cluster=T45 {"Solenoid #1"=FALSE, "Solenoid #2"=FALSE, "Air Pump On"=FALSE, "Flow(ml)"=0} ("element"), "Solenoid #1"=w294, "Solenoid #2"=w292, "Air Pump On"=w293, "Flow(ml)"=w298) -> (w297:T45)
                  n195 = Enqueue Element(queue=w302, element=w297) -> ()  [unwired: 2 in, 3 out]
                }
                event Value Change {
                  n196 = event-data() -> ("NewVal"=w311:bool)  [unwired: 1 in]
                  n197 = Unbundle By Name(w319) -> ("Queue Cluster.Pump"=w317:refnum<queue>, "Miscellaneous.Air Pump Controls"=w318:refnum<vi>)
                  n198 = property class="Clust (strict)"(reference=w318) -> ("Value"=w315:T35)  [unwired: 1 in, 2 out]
                  n199 = Unbundle By Name(w315) -> ("Air Pump On"=w312:bool, "Solenoid #1"=w310:bool, "Flow(ml)"=w314:u16)
                  n200 = Not(x=w311) -> (.not. x?=w309:bool)
                  n201 = Not(x=w310) -> (.not. x?=w307:bool)
                  n202 = Not(x=w312) -> (.not. x?=w308:bool)
                  n203 = Bundle By Name(cluster=T45 {"Solenoid #1"=FALSE, "Solenoid #2"=FALSE, "Air Pump On"=FALSE, "Flow(ml)"=0} ("element"), "Solenoid #1"=w307, "Solenoid #2"=w309, "Air Pump On"=w308, "Flow(ml)"=w314) -> (w313:T45)
                  n204 = Enqueue Element(queue=w317, element=w313) -> ()  [unwired: 2 in, 3 out]
                }
                event Value Change {
                  n205 = event-data() -> ()  [unwired: 1 in, 1 out]
                  n206 = Unbundle By Name(w334) -> ("Queue Cluster.Pump"=w332:refnum<queue>, "Miscellaneous.Air Pump Controls"=w333:refnum<vi>)
                  n207 = property class="Clust (strict)"(reference=w333) -> ("Value"=w323:T35)  [unwired: 1 in, 2 out]
                  n208 = call "Calculate Flow Rate.vi"("AirPump Controls"=w323) -> ("Flow Rate"=w322:i32)  [unwired: 10 in]
                  n209 = Unbundle By Name(w323) -> ("Air Pump On"=w329:bool, "Solenoid #1"=w328:bool, "Solenoid #2"=w327:bool)
                  n210 = Not(x=w329) -> (.not. x?=w326:bool)
                  n211 = Not(x=w328) -> (.not. x?=w325:bool)
                  n212 = Not(x=w327) -> (.not. x?=w324:bool)
                  n213 = Bundle By Name(cluster=T45 {"Solenoid #1"=FALSE, "Solenoid #2"=FALSE, "Air Pump On"=FALSE, "Flow(ml)"=0} ("element"), "Solenoid #1"=w325, "Solenoid #2"=w324, "Air Pump On"=w326, "Flow(ml)"=w322) -> (w330:T45)
                  n214 = Enqueue Element(queue=w332, element=w330) -> ()  [unwired: 2 in, 3 out]
                }
                event "Cluster 3.Pump Flow Rate": Value Change {
                  n215 = event-data() -> ("NewVal"=w340:u16)  [unwired: 1 in]
                  n216 = Unbundle By Name(w349) -> ("Queue Cluster.Pump"=w347:refnum<queue>, "Miscellaneous.Air Pump Controls"=w348:refnum<vi>)
                  n217 = property class="Clust (strict)"(reference=w348) -> ("Value"=w345:T35)  [unwired: 1 in, 2 out]
                  n218 = Unbundle By Name(w345) -> ("Air Pump On"=w343:bool, "Solenoid #1"=w342:bool, "Solenoid #2"=w341:bool)
                  n219 = Not(x=w343) -> (.not. x?=w339:bool)
                  n220 = Not(x=w342) -> (.not. x?=w338:bool)
                  n221 = Not(x=w341) -> (.not. x?=w337:bool)
                  n222 = Bundle By Name(cluster=T45 {"Solenoid #1"=FALSE, "Solenoid #2"=FALSE, "Air Pump On"=FALSE, "Flow(ml)"=0} ("element"), "Solenoid #1"=w338, "Solenoid #2"=w337, "Air Pump On"=w339, "Flow(ml)"=w340) -> (w344:T45)
                  n223 = Enqueue Element(queue=w347, element=w344) -> ()  [unwired: 2 in, 3 out]
                }
                event "Last Calibration.View Cal Details": Value Change {
                  n224 = event-data() -> ("CtlRef"=w354:refnum<vi>)  [unwired: 1 in]
                  n225 = property class="Bool (strict)"(reference=w354, "Value"=FALSE ("View Cal Details")) -> ()  [unwired: 1 in, 2 out]
                  n226 = global read "Globals.vi" "Calibration Coefficients"() -> (w352:T54[])
                  n227 = call "View and Edit Calibration Coefficients.vi"("Calibration Coefficients"=w352) -> ()  [unwired: 11 in]
                }
                event "Store_Cal": Value Change {
                  n228 = event-data() -> ("CtlRef"=w357:refnum<vi>)  [unwired: 1 in]
                  n229 = call "Save Copy of Cal Coefficients.vi"() -> ()  [unwired: 12 in]
                  n230 = property class="Bool (strict)"(reference=w357, "Value"=FALSE) -> ()  [unwired: 1 in, 2 out]
                }
                event "Record Button": Value Change {
                  n231 = event-data() -> ("NewVal"=w362:bool)  [unwired: 1 in]
                  n232 = call "Monitor Step 1.vi"("Daq Needed"=w361, "Record Button"=w362) -> ()  [unwired: 10 in]
                }
                event "Open Cal": Value Change {
                  n233 = event-data() -> ("CtlRef"=w369:refnum<vi>)  [unwired: 1 in]
                  n234 = property class="Bool (strict)"(reference=w369, "Value"=FALSE) -> ()  [unwired: 1 in, 2 out]
                  n235 = Unbundle By Name(w368) -> ("Queue Cluster.DAC Current"=w365:refnum<queue>, "Individuals.HomeMode"=w372:refnum<vi>)
                  n236 = call "Restore Copy of  Cal Coefficients.vi"() -> ("Calibration Coefficients"=w367:T54[])  [unwired: 11 in]
                  n237 = property class="TabCtl (strict)"(reference=w372, "Value"=T14."Initialising" ("HomeMode")) -> ()  [unwired: 1 in, 2 out]
                  n238 = for {
                    tunnel: w367 -> [w378] mode=indexing
                    tunnel: [w377] -> w366 mode=indexing
                    tunnel: [u8 0 ("element")] -> w373 mode=indexing
                    n239 = Unbundle By Name(w378) -> ("I_span"=w377:dbl)
                  }
                  n240 = global write "Globals.vi" "DAC Setting"(w373) -> ()
                  n241 = call "Set DAQ and Wait.vi"("Array"=w366, "Queue in"=w365) -> ()  [unwired: 10 in]
                }
                event "Run": Value Change {
                  n242 = event-data() -> ()  [unwired: 1 in, 1 out]
                }
                event "Cluster 9.Advanced": Value Change {
                  n243 = event-data() -> ("CtlRef"=w382:refnum<vi>)  [unwired: 1 in]
                  n244 = property class="Bool (strict)"(reference=w382, "Value"=FALSE) -> ()  [unwired: 1 in, 2 out]
                }
                event "Cluster 9.RTMode": Value Change {
                  n245 = event-data() -> ("NewVal"=w386:bool)  [unwired: 1 in]
                  n246 = call "Log.vi"("Daq Needed"=w385) -> ()  [unwired: 11 in]
                  n247 = call "GetBooleanSettings.vi"("Change Value"=w386, "Variable Name"="RTMode", "Mode"=T40."Change Item") -> ()  [unwired: 1 in, 4 out]
                  n248 = Boolean To (0,1)(Boolean=w386) -> (0, 1=→"CalTab":i16)
                }
                event "Cluster 9.Settings": Value Change {
                  n249 = event-data() -> ("CtlRef"=w396:refnum<vi>)  [unwired: 1 in]
                  n250 = Unbundle By Name(w393) -> ("Queue Cluster.Pump"=w392:refnum<queue>)
                  n251 = property class="Bool (strict)"(reference=w396, "Value"=FALSE) -> ()  [unwired: 1 in, 2 out]
                  n252 = Enqueue Element(queue=w392, element=T45 {"Solenoid #1"=TRUE, "Solenoid #2"=TRUE, "Air Pump On"=TRUE, "Flow(ml)"=0}) -> ()  [unwired: 2 in, 3 out]
                  n253 = call "GetBooleanSettings.vi"("Change Value"=FALSE, "Variable Name"="LoopActive", "Mode"=T40."Change Item") -> ("error out"=w400:errorcluster)  [unwired: 1 in, 3 out]
                }
                event "Cluster 9.Play Button": Value Change {
                  n254 = event-data() -> ("CtlRef"=w404:refnum<vi>, "NewVal"=w407:bool)  [unwired: 1 in]
                  n255 = Unbundle By Name(w408) -> ("Individuals.Sequence Stop"=w406:refnum<vi>, "Loflo.sequence"=w405:refnum<vi>)
                  n256 = case shown="True" w407 {
                    tunnel: w405 -> [_ w420]
                    tunnel: w404 -> [_ w418]
                    tunnel: w406 -> [_ w417]
                    frame False {
                    }
                    frame True {
                      n257 = call <vilib>:"Application Directory.vi"() -> ("Application Directory"=w414:path)
                      n258 = Strip Path(path=w414) -> (stripped path=w413:path)  [unwired: 1 out]
                      n259 = Build Path(base path=w413, name or relative path="SEQUENCES") -> (appended path=w411:path)
                      n260 = call "ReadFromSpreadsheet.vi"("transpose (no:F)"=TRUE, "File Prompt"="Open Sequence File", "file path"=w411) -> ("cancelled"=w422:bool, "first row"=w419:sgl[])  [unwired: 4 in, 3 out]
                      n261 = Not(x=w422) -> (.not. x?=w421:bool)
                      n262 = property class="Arr (strict)"(reference=w420, "Value"=w419) -> ()  [unwired: 1 in, 2 out]
                      n263 = property on="Property Node" class="Bool (strict)"(reference=w418, "Visible"=w422, "Value"=FALSE) -> ()  [unwired: 1 in, 2 out]
                      n264 = property on="Property Node" class="Bool (strict)"(reference=w417, "Visible"=w421) -> ()  [unwired: 1 in, 2 out]
                    }
                  }
                }
                event "Cluster 9.Sequence Stop": Value Change {
                  n265 = event-data() -> ("CtlRef"=w424:refnum<vi>, "NewVal"=w425:bool)  [unwired: 1 in]
                  n266 = Unbundle By Name(w426) -> ("Individuals.Play Button"=w427:refnum<vi>, "Loflo.sequence"=w428:refnum<vi>)
                  n267 = case shown="True" w425 {
                    tunnel: w428 -> [_ w435]
                    tunnel: w424 -> [_ w433]
                    tunnel: w427 -> [_ w432]
                    frame False {
                    }
                    frame True {
                      n268 = property on="Property Node" class="Bool (strict)"(reference=w432, "Visible"=TRUE) -> ()  [unwired: 1 in, 2 out]
                      n269 = property on="Property Node" class="Bool (strict)"(reference=w433, "Visible"=FALSE, "Value"=FALSE) -> ()  [unwired: 1 in, 2 out]
                      n270 = property class="Arr (strict)"(reference=w435, "Value"=i32[] []) -> ()  [unwired: 1 in, 2 out]
                    }
                  }
                }
                event "Off": Value Change {
                  n271 = event-data() -> ("CtlRef"=w441:refnum<vi>, "NewVal"=w442:bool)  [unwired: 1 in]
                  n272 = property class="Bool (strict)"(reference=w441, "Value"=FALSE) -> ()  [unwired: 1 in, 2 out]
                  n273 = Unbundle By Name(w443) -> ("Queue Cluster.Pump"=w439:refnum<queue>, "Individuals.Status Lights"=w447:refnum<vi>)
                  n274 = property class="Clust (strict)"(reference=w447) -> (reference out=w445:refnum<vi>, "Value"=w444:T3)  [unwired: 1 in, 1 out]
                  n275 = call "GetBooleanSettings.vi"("Change Value"=FALSE, "Variable Name"="LoopActive", "Mode"=T40."Change Item") -> ("error out"=w448:errorcluster)  [unwired: 1 in, 3 out]
                  n276 = Bundle By Name(cluster=w444, "Loop Active"=w442) -> (w446:T3)
                  n277 = Enqueue Element(queue=w439, element=T45 {"Solenoid #1"=TRUE, "Solenoid #2"=TRUE, "Air Pump On"=TRUE, "Flow(ml)"=0}) -> ()  [unwired: 2 in, 3 out]
                  n278 = property class="Clust (strict)"(reference=w445, "Value"=w446) -> ()  [unwired: 1 in, 2 out]
                }
                event "Cluster 9.Exit": Value Change {
                  n279 = event-data() -> ("CtlRef"=w455:refnum<vi>)  [unwired: 1 in]
                  n280 = property class="Bool (strict)"(reference=w455, "Value"=FALSE) -> ()  [unwired: 1 in, 2 out]
                  n281 = Two Button Dialog(message="Exit Button Pressed \nDo You Wish to Exit Application?" ("Window Title (\"\")"), 1:"No,Resume Setup", 2:"Yes Exit") -> (T button?=w456:bool)
                  n282 = case shown="True" w456 {
                    tunnel: w457 -> [_ w466]
                    frame False {
                      # "Setup Key Pressed"
                    }
                    frame True {
                      w465 = FALSE ("Change Value")
                      n283 = Unbundle By Name(w466) -> ("Queue Cluster.Pump"=w464:refnum<queue>, "Individuals.Status Lights"=w467:refnum<vi>)
                      n284 = property class="Clust (strict)"(reference=w467) -> (reference out=w469:refnum<vi>, "Value"=w470:T3)  [unwired: 1 in, 1 out]
                      n285 = Bundle By Name(cluster=w470, "Loop Active"=w465) -> (w468:T3)
                      n286 = property class="Clust (strict)"(reference=w469, "Value"=w468) -> ()  [unwired: 1 in, 2 out]
                      n287 = call "GetBooleanSettings.vi"("Change Value"=w465, "Variable Name"="LoopActive", "Mode"=T40."Change Item") -> ()  [unwired: 1 in, 4 out]
                      n288 = Enqueue Element(queue=w464, element=T45 {"Solenoid #1"=TRUE, "Solenoid #2"=TRUE, "Air Pump On"=TRUE, "Flow(ml)"=0}) -> ()  [unwired: 2 in, 3 out]
                    }
                  }
                }
                event "Cluster 7.Start": Value Change {
                  n289 = event-data() -> ("NewVal"=w476:bool)  [unwired: 1 in]
                  n290 = case shown="False" w476 {
                    tunnel: w475 -> [w480 w487]
                    frame False {
                      n291 = Unbundle By Name(w480) -> ("Temp Seq.Saving"=w479:refnum<vi>)
                      n292 = property class="Bool (strict)"(reference=w479, "Value"=FALSE) -> ()  [unwired: 1 in, 2 out]
                      n293 = global write "Globals.vi" "Ready to Log"(TRUE ("Ready to Log")) -> ()
                      n294 = call "GetBooleanSettings.vi"("Change Value"=FALSE, "Variable Name"="Start", "Mode"=T40."Change Item") -> ()  [unwired: 1 in, 4 out]
                    }
                    frame True {
                      n295 = call "Log.vi"("Daq Needed"=w487) -> ()  [unwired: 11 in]
                      n296 = call "GetBooleanSettings.vi"("Change Value"=TRUE, "Variable Name"="Start", "Mode"=T40."Change Item") -> ()  [unwired: 1 in, 4 out]
                    }
                  }
                }
                event "Waveforms": Value Change {
                  n297 = event-data() -> ("OldVal"=w494:T23, "NewVal"=w493:T23)  [unwired: 1 in]
                  n298 = Unbundle By Name(w496) -> ("DAQ.WFChart Refnum"=w495:refnum<vi>)
                  n299 = Equal?(x=w494, y=w493) -> (x = y?=w492:T55)
                  n300 = Cluster To Array(cluster=w492) -> (array=w491:bool[])
                  n301 = property class="WFChart (strict)"(reference=w495) -> ("DigDisps[]"=w490:refnum<vi>[])  [unwired: 1 in, 2 out]
                  n302 = for {
                    tunnel: w491 -> [w498] mode=indexing
                    tunnel: w490 -> [w497] mode=indexing
                    n303 = case shown="False" w498 {
                      tunnel: w497 -> [w505 _]
                      frame False {
                        w501 = T41."Enabled" ("y")
                        n304 = property class="DigNum"(reference=w505) -> (reference out=w504:refnum<vi>, "DisabledEnum"=w503:T41)  [unwired: 1 in, 1 out]
                        n305 = Equal?(x=w503, y=w501) -> (x = y?=w502:bool)
                        n306 = Select(t=T41."Disabled and Grayed Out", s=w502, f=w501) -> (s? t:f=w499:T41)
                        n307 = property class="DigNum"(reference=w504, "DisabledEnum"=w499) -> ()  [unwired: 1 in, 2 out]
                      }
                      frame True {
                      }
                    }
                  }
                }
                event "Insp Tank": Value Change {
                  n308 = event-data() -> ("NewVal"=w506:u8)  [unwired: 1 in, 5 out]
                  n309 = global write "Globals.vi" "Insp Tank"(w506) -> ()
                }
              }
              "Tab Control" <- w204
              n310 = call "GetBooleanSettings.vi"("error in"=w203, "Variable Name"="LoopActive") -> ("Set Value"=w205:bool)  [unwired: 2 in, 3 out]
              n311 = node-c288() -> ()  [unwired: 1 in, 1 out]
              "loop counter" <- w202
            }
            n312 = call "Threads.vi"("Daq Needed"=w184, "Offset Adjust"=w194, "DAQTasks in"=w191, "Pump Meter Use (mins) 2"=w192, "Digital Line Value"=w193) -> ()  [unwired: 6 in, 1 out]
            n313 = call "Get DAQ Offset and Set Start Values.vi"("Daq Needed"=w184) -> ("error out"=w189:errorcluster)  [unwired: 10 in]
            n314 = case shown="No Error" w189 {
              tunnel: w184 -> [w513 _]
              frame No Error {
                w519 = T41."Enabled" ("Disabled")
                n315 = property on="Tab Control" class="TabCtl (strict)"("DisabledEnum"=w519) -> ()  [unwired: 2 in, 2 out]
                n316 = property on="SetDac Button" class="Bool (strict)"("DisabledEnum"=w519) -> ()  [unwired: 2 in, 2 out]
                n317 = property on="Run" class="Bool"("DisabledEnum"=w519) -> ()  [unwired: 2 in, 2 out]
                n318 = call "GetBooleanSettings.vi"("Change Value"=TRUE, "Variable Name"="DAQsInitialized", "Mode"=T40."Change Item") -> ()  [unwired: 1 in, 4 out]
                n319 = Unbundle By Name(w513) -> ("Miscellaneous.RunTime Mode Settings  2"=w511:refnum<vi>, "Miscellaneous.DAQ Cluster 3"=w515:refnum<vi>)
                n320 = property class="Clust (strict)"(reference=w511, "Visible"=TRUE) -> ()  [unwired: 1 in, 2 out]
                n321 = property class="Clust (strict)"(reference=w515, "Visible"=TRUE) -> ()  [unwired: 1 in, 2 out]
              }
              frame Error {
              }
            }
            n322 = node-c288(w187) -> ()  [unwired: 1 out]
            n323 = local write "ExitProgram"(w190) -> ()
            n324 = call "GetBooleanSettings.vi"("Change Value"=w195, "Variable Name"="LoopActive", "Mode"=T40."Change Item") -> ()  [unwired: 1 in, 4 out]
          }
        }
      }
    }
  }
